vi "AlliGator Phasor Graph Actions.vi"(0 "AlliGator Q Elements in":T6[](array[typedef]), 1 "VI in":refnum<vi>, 2 "Script in":bool, 5 "Data Value Reference in":refnum<data-value>, 7 "AlliGator Q Event in":T7=enum."GUI:Idle", 9 "Data":variant, 11 "error in (no error)":errorcluster, 12 "AlliGator Ctrl Refnums":T8) -> (3 "Script out":bool, 4 "AlliGator Q Elements out":T6[](array[typedef]), 6 "Data Value Reference out":refnum<data-value>, 10 "[Notebook Message]":T1[](array[typedef]) {"Message Style"."Font Size" min=6.0 step=1.0}, 15 "error out":errorcluster)   [LabVIEW 2021, in "AlliGator Action Engine.lvlib"]
doc: "Processes AlliGator phasor graph-related actions."
uses:
  AlliGator Action Engine.lvlib
  Internal Variables/AlliGator Internal Variables v2.ctl
  <vilib>/vision/Image Controls.llb/IMAQ Image.ctl
  Internal Variables/AlliGator Gate Image Set.ctl
  Files/AlliGator FLI Dataset Type.ctl
  Files/AlliGator Data Series Type.ctl
  Dual-Channel Datasets/AlliGator Dataset Channel.ctl
  Settings/AlliGator Gate Arithmetic.ctl
  Source Image/AlliGator Displayed Image.ctl
  Image/Named ROI Description.ctl
  Phasor Graph/AlliGator Decay Metadata v3.ctl
  Decay Analysis/Decay Preprocessing/AlliGator Decay Background Subtraction Info.ctl
  Decay Analysis/Decay Preprocessing/AlliGator Baseline Subtraction Method.ctl
  Graphs/XY Graph/XY Graph Plot Shift Parameters.ctl
  Graphs/XY Graph/XY Graph Plot Shift Method.ctl
  Decay Analysis/Decay Preprocessing/AlliGator Decay Extrapolation Parameters.ctl
  Phasor/Calibration Phasor (m, phi).ctl
  Phasor/Phasor Reference Series.ctl
  Phasor/Phasor Calibration Map v2.ctl
  Phasor/Phasor (g, s).ctl
  Phasor Graph/AlliGator Raw Phasor Plot Data v5.ctl
  Phasor/Phasor Standard Deviation Options.ctl
  Phasor Plot/AlliGator Phasor Multi-Harmonic Data.ctl
  Phasor/Phasor Harmonic Data.ctl
  Decay Fit Parameter Map/AlliGator Decay Fit Options & Parameters v3.ctl
  Fits/IRF(X)PSED/Decay Fit Options v3.ctl
  Fits/Decay Convolution/Decay Model.ctl
  Fits/Residual Type.ctl
  Fits/IRF(X)PSED/Fit Weights Type.ctl
  Fits/Non-linear Fitting Method v2.ctl
  Fits/Fit Calculation Method.ctl
  Fits/Non-linear Fitting Algorithm.ctl
  Decay Analysis/Decay Fit/AlliGator Decay Fit Parameter Constraints 2.ctl
  Fits/IRF(X)PSED/Decay Fit Parameters In List.ctl
  Fits/IRF(X)PSED/MLE Baseline Offset Type.ctl
  Decay Analysis/Decay Preprocessing/AlliGator Decay Preprocessing Parameters.ctl
  Fits/IRF(X)PSED/Decay Fit Parameters & Derived Quantities List v2.ctl
  Fits/IRF(X)PSED/Decay Fit Result Constraint.ctl
  Decay Fit Parameter Map/AlliGator Parameter Maps Data.ctl
  AlliGator Q Event.ctl
  GUI/AlliGator Ctrl Refnums.ctl
  GUI/AlliGator Other Ctrl Refnums.ctl
  GUI/AlliGator State Indicator.ctl
  GUI/AlliGator Main Window Tabs.ctl
  GUI/AlliGator Phasor Plot Ctrl Refnums.ctl
  GUI/AlliGator Phasor Graph Ctrl Refnums.ctl
  Phasor/Phasor Calibration Type.ctl
  GUI/AlliGator Dataset Ctrl Refnums.ctl
  GUI/AlliGator Registered Events Ctrl Refnums.ctl
  GUI/AlliGator Image Histogram Control Refnums.ctl
  Histograms/Linear Histogram Options.ctl
  Histograms/Histogram Bin Option.ctl
  Histograms/Histogram Bin Position.ctl
  Decay Fit Parameter Map/AlliGator Decay Fit Map Control Refnums.ctl
  Parameter Map/AlliGator Parameter Map Control Refnums.ctl
  AlliGator Q Element.ctl
  Notebook/Notebook Message Object.ctl
  Rich Text Box/Text Formatting.ctl
  Rich Text Box/Text Colors.ctl
  Rich Text Box/Text Style.ctl
  Rich Text Box/Text Alignment.ctl
  Graphs/XY Graph/XY Graph Mouse Click Event Data.ctl
  Graphs/XY Graph/XY Graph Refnum.ctl
  <vilib>/Utility/miscctls.llb/LVPoint32TypeDef.ctl
  Graphs/XY Graph/XY Graph Selected Plot Info.ctl
  Phasor Graph/AlliGator Raw Phasor Plot Array Action.ctl
  Alligator Elements Order in Action Stack.ctl
  Rich Text Box/Text Format List.ctl
  Graphs/XY Graph/New Plot Information.ctl
  Graphs/Plot Scales.ctl
  Graphs/LabVIEW Plot Interpolation.ctl
  Graphs/Plot Point Style.ctl
  Globals, Variables, Constants/AlliGator Variables List.ctl
  Phasor Graph/AlliGator Phasor Plot Scatter Plot Parameters.ctl
  Phasor Graph/AlliGator Phasor Graph Parameter List.ctl
  Phasor Ratio/AlliGator Phasor Reference Data.ctl
  Phasor/Phasor (m, phi).ctl
  da8c548c-3fe3-4ac5-84e2-54aef6c91d4f.vi
  Graphs/Get Plot at Mouse Click (XY Graph)/Get Plot at Mouse Click [AAC].vi
  AlliGator Add Single Action to Stack.vi
  AlliGator Add Action Array to Stack.vi
  Variant/Variant to Data/Variant to Boolean.vi
  Variant/Variant to Data/Variant to Path.vi
  Variant/Variant to Data/Variant to [Path].vi
  Arrays/Signed Array Index.vi
  Variant/Variant to Data/Variant to I32.vi
  <vilib>/Utility/error.llb/Error Cluster From Error Code.vi
  Variant/Variant to Data/Variant to U32.vi
  <userlib>/_OpenG.lib/array/array.llb/Filter 1D Array with Scalar (I32)__ogtk.vi
  <vilib>/ErrorRing/Error Ring.xnode
  Graphs/Graphs.lvlib
  Variant/Variant to Data/Variant to Data.lvlib
  Phasor Graph/AlliGator Phasor Graph.lvlib
  Internal Variables/AlliGator Internal Variables.lvlib
  GUI/GUI.lvlib
  Phasor/Phasor.lvlib
  Graphs/XY Graph/XY Graph Add-Ons.lvlib
  Phasor Ratio/AlliGator Phasor Ratio.lvlib
  Strings/Strings.lvlib
  <userlib>/_OpenG.lib/array/array.llb/openg_array.lvlib
  Scripts/AlliGator Scripts.lvlib
  Source Image/AlliGator Source Image.lvlib
  Files/AlliGator Files.lvlib
  Settings/AlliGator Settings.lvlib
  Sound/Sound.lvlib
  Error/Error.lvlib
  Globals, Variables, Constants/AlliGator Globals, Variables & Constants.lvlib
  Phasor Calibration/AlliGator Phasor Calibration.lvlib
  Notebook/Notebook.lvlib
  Image/Image.lvlib
  Decay Analysis/Decay Preprocessing/AlliGator Decay Preprocessing.lvlib
  Phasor Plot/AlliGator Phasor Plot.lvlib
  Fits/Fits.lvlib
  Decay Analysis/Decay Fit/AlliGator Decay Fit.lvlib
  Decay Fit Parameter Map/AlliGator Decay Fit Parameter Map.lvlib
  GUI/AlliGator GUI.lvlib
  Rich Text Box/Rich Text Box.lvlib
  Dual-Channel Datasets/AlliGator Dual-Channel Datasets.lvlib
  Histograms/Histogram Window.lvlib
  Parameter Map/AlliGator Parameter Map.lvlib
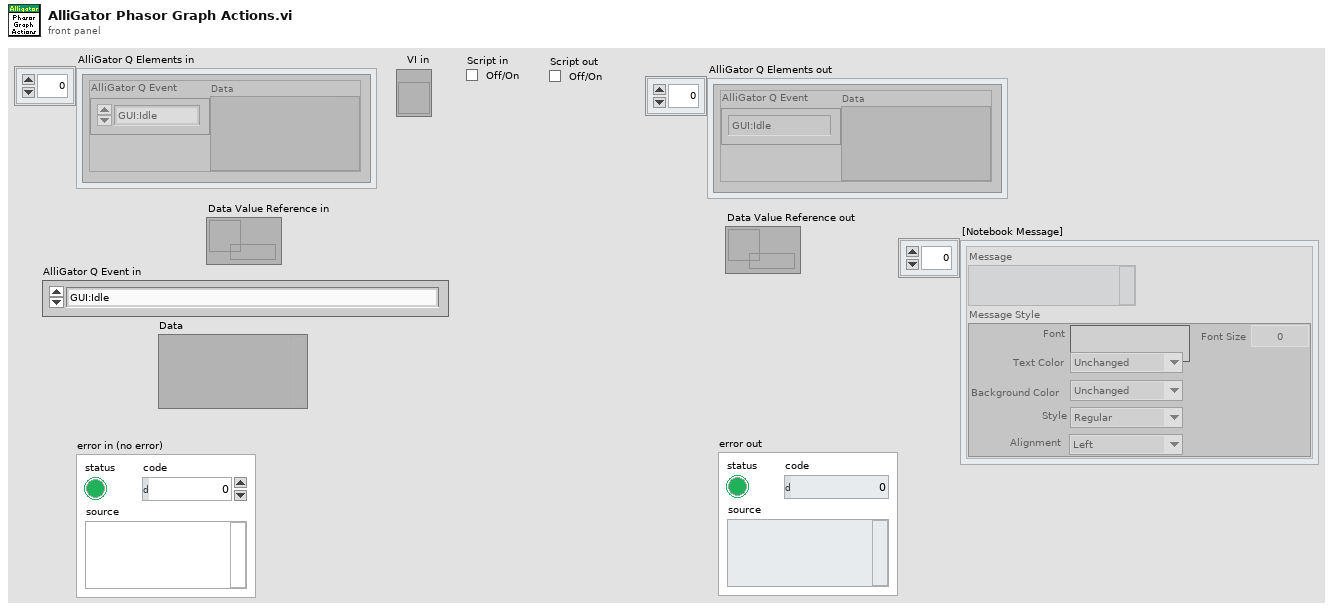
[diagram p1: front panel]
types:
  T1 = typedef "Notebook.lvlib/Notebook Message Object.ctl" = cluster{"Message":string, "Message Style":T2}
  T2 = typedef "Rich Text Box.lvlib/Text Formatting.ctl" = cluster{"Font":string, "Text Color":T3, "Background Color":T3, "Style":T4, "Font Size":dbl, "Alignment":T5}
  T3 = typedef "Rich Text Box.lvlib/Text Colors.ctl" = enum16{"Unchanged", "Black", "Blue", "Cyan", "Maroon", "Gray", "Violet", "Green", "Light Green", "Orange", "Yellow", "Magenta", "Red", "White"}
  T4 = typedef "Rich Text Box.lvlib/Text Style.ctl" = enum16{"Regular", "Bold", "Italic", "Underline", "Strikeout"}
  T5 = typedef "Rich Text Box.lvlib/Text Alignment.ctl" = enum16{"Left", "Right", "Center"}
  T6 = typedef "AlliGator Action Engine.lvlib/AlliGator Q Element.ctl" = cluster{"AlliGator Q Event":T7, "Data":variant}
  T7 = typedef "AlliGator Action Engine.lvlib/AlliGator Q Event.ctl" = enum16{"---- Files ----", "Files:Set Batch Export Files To Save", "Files:Set Dataset Loading & Pre-processing Options", "Files:Check #Frames in Dataset", "Files:Increment Frame Index", "Files:Open Mask Image", "Files:Open White Light Image", "Files:Open Single Dataset", "Files:New Folder of Folders Selected", "Files:Load File (all Types)_Scriptable", "Files:Move Flattened Series to Folders Series", "Files:Select Folder", "Files:Load FLI Dataset", "Files:Load Swiss SPAD 1 Dataset", "Files:Load Swiss SPAD 2 Dataset", "Files:Load .sdt FLI Dataset", "Files:Load .ptu FLI Dataset", "Files:Load .bin FLI Dataset", "Files:Load Single Gate Image Folder", "Files:Load I/m/phi Dataset (deprecated)", "Files:Load Single Image", "Files:Subtract Background File", "Files:Export FLI Dataset", "Files:Load HDF5 FLI Dataset", "Files:Set Destination File Path", "Files:Save Mask Image", "Files:Batch Conversion", "Files:New Folder Selected", "Files:Close FLI Dataset", "Files:Close FLI Dataset Series", "Files:Close White Light Image", "Files:Close Mask Image", "---- FLI Dataset ----", "FLI Dataset:Channel Arithmetic", "FLI Dataset:Export Average Lifetime Map as ASCII", "FLI Dataset:Export User-Defined Quantity Map as ASCII", "FLI Dataset:Python Function FLI Dataset Event", "FLI Dataset:ROI Analysis", "FLI Dataset:Tilted Logistic Square Gated IRF Characteristics Map", "FLI Dataset:Logistic Square Gated IRF Characteristics Map", "FLI Dataset:Square Gated IRF Characteristics Map", "FLI Dataset:Multi-ROI Single-Pixel Phasor Analysis", "FLI Dataset:Multi-ROI Single-Pixel NLSF Analysis", "FLI Dataset:All ROIs IRF Extraction", "FLI Dataset:All ROIs Decay Fit Non-Interactive (Fast + Individual IRF)", "FLI Dataset:All ROIs Phasor Analysis", "FLI Dataset:All ROIs Decay Fit", "FLI Dataset:Fluorescence Decay Statistics", "FLI Dataset:Update Decay Statistics Graph", "FLI Dataset:Get Decay from ROI", "FLI Dataset:All ROIs Average Lifetimes", "FLI Dataset:Save/Load Local IRFs", "FLI Dataset:Clear Local IRFs", "FLI Dataset:Phasor Calibration Maps (# Gates Series) Script", "FLI Dataset:Calibrated Phasor Map Series", "---- FLI Dataset Series ----", "FLI Dataset Series:Sum All Datasets in Series", "FLI Dataset Series:Add Dataset to Accumulated Dataset", "FLI Dataset Series:Display Accumulated Dataset", "FLI Dataset Series:Clear Dataset Series Sum", "FLI Dataset Series:Time-Series Analysis (NLSF)", "FLI Dataset Series:Time-Series Analysis (Phasor)", "---- Image ----", "Image:Update Image Profile Plots", "Image:Image Histogram Cursor Move", "Image:Image Histogram", "Image:Image Contrast", "Image:Set Image Histogram Cursor Move Flag", "Image:Clear Image Overlay", "Image:Use ROI as Search Area", "Image:Set ROI Diameter", "Image:Save Image Data as TIFF", "Image:Save Displayed Image with Overlay", "Image:Save Image Overlay Only", "Image:Save Image as Hot Pixel Mask", "Image:Change Source Image Color Palette", "Image:Copy Image to Clipboard", "Image:Source Image ROI Selection", "Image:Delete All ROIs", "Image:Delete All Unselected ROIs", "Image:Delete ROI", "Image:Merge All ROIs", "Image:Store ROI", "Image:Source Image ROI Storage", "Image:Export ROI Description to Notebook", "Image:Save ROI", "Image:Load ROI", "Image:Paste ROI Definition", "Image:Clear ROI", "Image:Identify ROIs in Mask Image", "Image:Create Complementary ROI", "Image:Create Contour ROI", "Image:Create ROI(s) from Pixels with Peak above Min_Scriptable", "Image:Create ROI(s) from Pixels with Intensity above Min_Scriptable", "Image:Compute ROI Statistics", "Image:Delete ROI(s) based on ROI Characteristics", "Image:Create ROI Grid", "Image:ROI to Individual Pixel ROIs", "Image:Python Function Source Image Event", "Image:Show Phasor Calibration Map ROI Centers", "Image:Convert ROI to Mask Image", "Image:Mouse Move", "Image:Mouse Up", "Image:Set Source Image Mouse Move Flag", "Image:Add Scale Bar Overlay", "Image:Delete Existing ROIs Option", "Image:Overlay ROI Median", "Image:Check Current ROI", "Image:Update True Pixel Value", "---- Decay ----", "Decay:Clear IRF/Reference Plot", "Decay:Add Decay to Graph", "Decay:Smoothen Plot", "Decay:Smoothen Plot Tail", "Decay:Average Selected Plots", "Decay:Extract IRF", "Decay:Optimal IRF Extraction", "Decay:Threshold IRF", "Decay:Fit to Model IRF", "Decay:Fit IRF to Square Gate", "Decay:Fit IRF to Logistic Square Gate", "Decay:Fit IRF to Tilted Logistic Square Gate", "Decay:Create Bounding Cursors Set", "Decay:Export Bounding Cursors Definition to Notebook", "Decay:Denoise Plot", "Decay:Compute Cumulative Function", "Decay:Use as Reference Decay", "Decay:Show Reference Decay/IRF", "Decay:Extrapolate Decay", "Decay:Create Head & Tail Bounding Cursors", "Decay:Store Cursor-defined Head & Tail Fractions", "Decay:Rebin Plot", "Decay:1-Normalize Decay", "Decay:[0-1]-Normalize Plot", "Decay:Straighten Decay", "Decay:Shift Decay", "Decay:Fold Decay", "Decay:Fit Decay", "Decay:Global Fit of Selected Decays", "Decay:Post Global Fit Script", "Decay:Add Global Fit Parameters to Graph", "Decay:Add Decay Parameter(s) to Plot (Graph)", "Decay:Export Decay to Phasor Graph", "Decay:Compute Average Lifetime", "Decay:Plot Convolution", "Decay:Graph Tip Strip Update", "---- Decay Statistics ----", "Decay Statistics:Tip Strip Update", "---- Intensity Time Trace ----", "Intensity Time Trace:Use File Timestamp", "Intensity Time Trace:Load Intensity Corrections File", "Intensity Time Trace:Clear Intensity Corrections File", "Intensity Time Trace:Tip Strip Update", "---- Phasor Plot ----", "Phasor Plot:Build Phasor Plot", "Phasor Plot:Change Phasor Plot Color Palette", "Phasor Plot:Adjust Phasor Plot Display Range", "Phasor Plot:Highlight Image ROI in Phasor Plot", "Phasor Plot:Save Phasor Plot Image with Overlay", "Phasor Plot:Export Complex Phasor Map", "Phasor Plot:Export Phasor Ratio Map", "Phasor Plot:Export Average Lifetime Map", "Phasor Plot:Compute Phase Lifetime Histogram", "Phasor Plot:Compute Phasor Ratio Histogram", "Phasor Plot:Compute Phase Lifetime vs Intensity Scatter Plot", "Phasor Plot:Weber 2-Component Decomposition", "Phasor Plot:Update Phasor Color Map Vertices", "Phasor Plot:Clear Phasor Overlay", "Phasor Plot:Use Segment Extremities as References", "Phasor Plot:Use UC/Segment Intersections as References", "Phasor Plot:Use UC/Principal Axis Intersections as References", "Phasor Plot:Use UC/Linear Fit Intersections as References", "Phasor Plot:Update Phasor Plot Reference", "Phasor Plot:Show Local Phasor Info in Phasor Plot", "Phasor Plot:Update Phasor Plot State", "Phasor Plot:Phasor Plot ROI Storage", "Phasor Plot:Phasor Plot ROI Selection", "Phasor Plot:Python Function Phasor Plot Event", "Phasor Plot:Overlay Phasor ROI, Ratio or Map in Source Image", "Phasor Plot:Compute Decay of Selected Phasors", "Phasor Plot:Phasor at Image Pixel", "Phasor Plot:Mouse Move", "Phasor Plot:Mouse Up", "Phasor Plot:Display Range Mouse Move", "Phasor Plot:Set Mouse Move Flag", "Phasor Plot:Update True Phasor Plot Value", "---- Phasor Graph ----", "Phasor Graph:Get Phasor Value", "Phasor Graph:Create New Phasor Plot Dialog", "Phasor Graph:Update Last Phasor Value", "Phasor Graph:Update Phasor (m, phi)", "Phasor Graph:Remove Single Phasor from Plot", "Phasor Graph:Add Single Phasor to Plot", "Phasor Graph:Remove Phasor Plot", "Phasor Graph:Remove Selected Phasor Plots", "Phasor Graph:Clear Phasor Data", "Phasor Graph:Clear Phasor Graph", "Phasor Graph:Cursor Move", "Phasor Graph:Draw Cursor Connecting Line", "Phasor Graph:Clear Cursor Connecting Line", "Phasor Graph:Find UC Intersection", "Phasor Graph:Use UC/Cursor-Defined Line Intersections", "Phasor Graph:Use Selected Plots Fitted Line/UC Intersections", "Phasor Graph:Use Selected Plots Principal Axis/UC Intersections", "Phasor Graph:Show Single Phasor", "Phasor Graph:Save Single Phasor Plot", "Phasor Graph:Save All Phasor Plots", "Phasor Graph:Load Phasor Plot(s)", "Phasor Graph:Phasor Multiplication", "Phasor Graph:Compute Average Phasor", "Phasor Graph:Compute Multiple Average Phasors (Selected Plots)", "Phasor Graph:Export Single Phasor Plot Phase Lifetimes", "Phasor Graph:Parameter 2 vs Parameter 1 Scatter Plot", "Phasor Graph:Use Cursor n Location", "Phasor Graph:Set Reference n to Current Phase Lifetime Value", "Phasor Graph:Set Reference n to Lifetime Value", "Phasor Graph:Set Cursor n Location", "Phasor Graph:Save Phasor Graph Image", "Phasor Graph:Update SEPL Plot", "Phasor Graph:Export Single Phasor Plot Data", "Phasor Graph:Export Selected Phasor Plots Data", "Phasor Graph:Python Function Phasor Graph Event", "Phasor Graph:Tip Strip Update", "---- Calibration ----", "Calibration:Set Calibration Type", "Calibration:Load/Save Phasor Calibration", "Calibration:Load/Save Phasor Calibration Series", "Calibration:Load/Save Phasor Calibration Map", "Calibration:Use as Calibration", "Calibration:Compute Optimal Calibration from Phasor References", "Calibration:Clear Phasor Calibration", "Calibration:Single Phasor Calibration Information", "Calibration:Use as Calibration Series", "Calibration:Use as Calibration Map", "Calibration:Clear Calibration Series", "Calibration:Phasor Calibration Series Information", "Calibration:Clear Calibration Map", "Calibration:Phasor Calibration Map Information", "Calibration:Apply Phasor Calibration", "Calibration:Update Single Plot Calibration", "Calibration:Update Multiple Plots Calibration", "Calibration:Clear Single Plot Calibration", "Calibration:Clear All Plots Calibrations", "Calibration:Clear Plot(s) Calibration(s)?", "---- Phasor Ratio ----", "Phasor Ratio:Clear Reference n", "Phasor Ratio:Toggle Selected Plot(s)  Lock to Reference 1", "Phasor Ratio:Use as Reference n", "Phasor Ratio:Send Reference n to Notebook", "Phasor Ratio:Toggle Selected Plot(s)  Lock to Reference 2", "Phasor Ratio:Compute Phasor Ratio at Mouse Location", "Phasor Ratio:Compute Phasor Plot's Average Phasor Ratio", "Phasor Ratio:Compute Time-Series Phasor Ratios", "Phasor Ratio:Fit Line to Phasor Ratio Plot", "Phasor Ratio:Save References", "Phasor Ratio:Load References", "Phasor Ratio:Update Phasor Reference 1", "Phasor Ratio:Update Phasor Reference 2", "Phasor Ratio:Move Cursor n to Reference n", "Phasor Ratio:Use as Phasor Reference 1 Lifetime", "Phasor Ratio:Use as Phasor Reference 2 Lifetime", "Phasor Ratio:Export Phasor Ratio Map as ASCII", "Phasor Ratio:Tip Strip Update", "---- Lifetime & Other Parameters Graph ----", "Lifetime:Compute Sliced Mean, SDV and CV Plots", "Lifetime:Plot Decay Shifts", "Lifetime:Plot Histogram", "---- Decay Fit Parameter Map ----", "Decay Fit Parameter Map:Export ROI NLSF Data as ASCII", "Decay Fit Parameter Map:Set Decay Fit Parameter Map Selection", "Decay Fit Parameter Map:Build Decay Fit Parameter Map", "Decay Fit Parameter Map:Change Decay Fit Parameter Map Color Palette", "Decay Fit Parameter Map:Export Decay Fit Parameter Map Data as ASCII", "Decay Fit Parameter Map:Export All Decay Fit Parameter Maps Data as ASCII", "Decay Fit Parameter Map:Selected Parameter Scatterplot", "Decay Fit Parameter Map:Parameter 2 vs Parameter 1 Scatterplot", "Decay Fit Parameter Map:Save Decay Fit Parameter Map Image", "Decay Fit Parameter Map:Save-Load IRFs & Fit Data", "Decay Fit Parameter Map:Update Local Decay Plots", "Decay Fit Parameter Map:Python Function Decay Fit Parameters Map Event", "Decay Fit Parameter Map:Overlay Decay Fit Parameter Map in Source Image", "Decay Fit Parameter Map:Selected Parameter vs Intensity Scatterplot", "Decay Fit Parameter Map:Mouse Up", "Decay Fit Parameter Map:Mouse Move", "Decay Fit Parameter Map:Display Range Mouse Move", "Decay Fit Parameter Map:Change Map Resolution", "Decay Fit Parameter Map:Variance Significance Maps", "Decay Fit Parameter Map:Fit Result Constraints Window", "---- Parameter Map ----", "Parameter Map:Export ROI Parameters Data as ASCII", "Parameter Map:Delete Parameter Map Set", "Parameter Map:Update Parameter List", "Parameter Map:Build Parameter Map", "Parameter Map:Change Parameter Map Color Palette", "Parameter Map:Export Parameter Map Data as ASCII", "Parameter Map:Export All Parameter Maps Data as ASCII", "Parameter Map:Selected Parameter Scatterplot", "Parameter Map:Parameter 2 vs Parameter 1 Scatterplot", "Parameter Map:Selected Parameter vs Intensity Scatterplot", "Parameter Map:Save Parameter Map Image", "Parameter Map:Save-Load IRFs & Parameter Maps (TODO)", "Parameter Map:Set Parameter Map Selection", "Parameter Map:Python Function Parameter Map Event", "Parameter Map:Overlay Parameter Map in Source Image", "Parameter Map:Update Local Decay Plots", "Parameter Map:Mouse Up", "Parameter Map:Mouse Move", "Parameter Map:Display Range Mouse Move", "---- Generic Graph ----", "Generic Graph:Generic XY Graph Event", "Generic Graph:Python Function XY Graph Event", "Generic Graph:New Plot", "Generic Graph:Save Plot", "Generic Graph:XY Plot Histogram", "Generic Graph:Set XY Graph Plot Name", "Generic Graph:Set Last Cursor Style", "Generic Graph:Tip Strip Update", "---- GUI ----", "GUI:Start Script", "GUI:Type of Displayed Image Changed", "GUI:Gate Image Slide Changed", "GUI:Show Busy Icon", "GUI:Show Busy Icon & Abort Button", "GUI:Hide Busy Icon", "GUI:Hide Busy Icon & Abort Button", "GUI:Abort", "GUI:End Script", "GUI:Start Timing", "GUI:End Timing", "GUI:Set State Indicator", "GUI:Send Parameters JSON Strings to Clipboard", "GUI:Set Gate Step", "GUI:Idle", "GUI:Initialization", "GUI:Quit", "GUI:Increment Dataset Index", "GUI:Set Dataset Index to -1", "GUI:Time Series Slider Moved", "GUI:Time Series Slider Changed", "GUI:Toggle Playback or Loop", "GUI:Playback Script", "GUI:Set Phasor Frequency", "GUI:Open Window", "GUI:Start Test Script", "GUI:End Test Script", "GUI:Set Verbose Mode", "GUI:Set Verbose Settings Mode", "DEBUG"}
  T8 = typedef "AlliGator GUI.lvlib/AlliGator Ctrl Refnums.ctl" = cluster{"Other AlliGator Ctrl Refnums":T9, "Phasor Plot Ctrl Refnums":T10, "Phasor Graph Ctrl Refnums":T11, "Dataset Control Refnums":T12, "Registered Events Ctrl Refnums":T13, "Image Histogram Ctrl Refnums":T14, "Decay Fit Map Ctrl Refnums":T15, "Parameter Map Ctrl Refnums":T16}
  T9 = typedef "AlliGator GUI.lvlib/AlliGator Other Ctrl Refnums.ctl" = cluster{"State Indicators":refnum<vi>, " Progress Bar":refnum<vi>, "Decay Graph Active":refnum<vi>, "Decay Statistics Bin":refnum<vi>, "Time Step":refnum<vi>, "Use File Timestamp":refnum<vi>, "Tab Control":refnum<vi>, "CPU":refnum<vi>, "Abort Fit":refnum<vi>, "Dataset File/Folder Path":refnum<vi>, "Abort ROI Creation":refnum<vi>, "Event LED":refnum<vi>, "Dataset File/Folder Path 2":refnum<vi>, "Dataset File/Folder Path 3":refnum<vi>, "Dataset File/Folder Path 4":refnum<vi>, "Dataset File/Folder Path 5":refnum<vi>, "Dataset File/Folder Path 6":refnum<vi>, "Dataset File/Folder Path 7":refnum<vi>, "Dataset File/Folder Path 8":refnum<vi>, "Dataset File/Folder Path 9":refnum<vi>, "Dataset File/Folder Path 10":refnum<vi>, "Dataset File/Folder Path 11":refnum<vi>}
  T10 = typedef "AlliGator GUI.lvlib/AlliGator Phasor Plot Ctrl Refnums.ctl" = cluster{"Phasor Ratio":refnum<vi>, "Modulus Lifetime":refnum<vi>, "Phasor at cursor (m, phi)":refnum<vi>, "Phase Lifetime":refnum<vi>, "Phasor at cursor (g, s)":refnum<vi>, "Phasor Plor Average Lifetime":refnum<vi>, "Phasor Plot Active":refnum<vi>, "Save Phasor Plot":refnum<vi>, "Image Overlay Color":refnum<vi>, "Phasor Plot Color Scale":refnum<vi>, "Reference 1 Button":refnum<vi>, "Reference 2 Button":refnum<vi>, "True Phasor Plot Value":refnum<vi>}
  T11 = typedef "AlliGator GUI.lvlib/AlliGator Phasor Graph Ctrl Refnums.ctl" = cluster{"Phasor Ratio":refnum<vi>, "Modulus Lifetime":refnum<vi>, "Phasor at cursor (m, phi)":refnum<vi>, "Phase Lifetime":refnum<vi>, "Phasor at cursor (g, s)":refnum<vi>, "Phasor Graph Average Lifetime":refnum<vi>, "Phasor Graph Active":refnum<vi>, "Save Phasor Graph":refnum<vi>, "Phasor Frame Slide":refnum<vi>, "Single Step Phasor":refnum<vi>, "Calibration Type":refnum<vi>, "Show Line":refnum<vi>, "Phase Lifetime 1":refnum<vi>, "Phase Lifetime 2":refnum<vi>, "Phasor Graph Frequency":refnum<vi>, "Phasor Reference 1 Control":refnum<vi>, "Phasor Reference 2 Control":refnum<vi>, "Calibration Lifetime":refnum<vi>, "Phase Lifetime SDV":refnum<vi>, "Average Lifetime SDV":refnum<vi>, "Phasor Ratio SDV":refnum<vi>, "Modulus Lifetime SDV":refnum<vi>}
  T12 = typedef "AlliGator GUI.lvlib/AlliGator Dataset Ctrl Refnums.ctl" = cluster{"Current Data":refnum<vi>, "Gate Image Slide":refnum<vi>, "Time Point Slide":refnum<vi>, "Current Time Stamp":refnum<vi>, "Save Image":refnum<vi>, "Displayed Image":refnum<vi>, "Overlay Mode":refnum<vi>, "Phasor Overlay Color":refnum<vi>, "Image Color Scale":refnum<vi>, "Use ROI as Search Area":refnum<vi>, "Source Image ROI Color":refnum<vi>, "True Pixel Value":refnum<vi>}
  T13 = typedef "AlliGator GUI.lvlib/AlliGator Registered Events Ctrl Refnums.ctl" = cluster{"Time Point Slider":refnum<vi>, "Phasor Plot Display Range":refnum<vi>, "Decay Graph":refnum<vi>, "Decay Statistics Graph":refnum<vi>, "Intensity Time Trace":refnum<vi>, "Phasor Graph":refnum<vi>, "Phasor Ratio Graph":refnum<vi>, "Lifetime Graph":refnum<vi>, "Phasor Plot Display":refnum<vi>, "Source Image Display":refnum<vi>, "Decay Fit Parameter Map Display Range":refnum<vi>, "Decay Fit Parameter Map Display":refnum<vi>, "Parameter Map Display Range":refnum<vi>, "Parameter Map Display":refnum<vi>, "Phasor Plot Display Range":refnum<vi>}
  T14 = typedef "AlliGator GUI.lvlib/AlliGator Image Histogram Control Refnums.ctl" = cluster{"Image Histogram":refnum<vi>, "Image Histogram Options":refnum<vi>, "Image Histogram Active":refnum<vi>, "Image Histogram Upper Percentile":refnum<vi>, "Image Histogram Lower Percentile":refnum<vi>, "Auto-Adjust Contrast":refnum<vi>}
  T15 = typedef "AlliGator Decay Fit Parameter Map.lvlib/AlliGator Decay Fit Map Control Refnums.ctl" = cluster{"Decay Fit Parameter Map Color Scale":refnum<vi>, "Decay Fit Parameter":refnum<vi>, "Max Parameter":refnum<vi>, "Min Parameter":refnum<vi>, "Decay Fit Parameter Map Display":refnum<vi>, "Decay Fit Parameter Map Display Range":refnum<vi>, "Decay Parameter Map X":refnum<vi>, "Decay Parameter Map Y":refnum<vi>, "Decay Parameter Map Value":refnum<vi>}
  T16 = typedef "AlliGator Parameter Map.lvlib/AlliGator Parameter Map Control Refnums.ctl" = cluster{"Parameter Map Color Scale":refnum<vi>, "Map Parameter":refnum<vi>, "Max Parameter":refnum<vi>, "Min Parameter":refnum<vi>, "Parameter Map Display":refnum<vi>, "Parameter Map Display Range":refnum<vi>, "Parameter Map Set":refnum<vi>, "Parameter Map X":refnum<vi>, "Parameter Map Y":refnum<vi>, "Parameter Map Value":refnum<vi>}
  T17 = typedef "XY Graph Add-Ons.lvlib/XY Graph Selected Plot Info.ctl" = cluster{"Multiplot XY Graph":T18, "Mouse Coordinates":T19, "Plot Index":i32}
  T18 = typedef "XY Graph Add-Ons.lvlib/XY Graph Refnum.ctl" = refnum<vi>
  T19 = typedef "LVPoint32TypeDef.ctl" = cluster{"Horizontal":i32, "Vertical":i32}
  T20 = typedef "XY Graph Add-Ons.lvlib/XY Graph Mouse Click Event Data.ctl" = cluster{"Multiplot XY Graph":T18, "Mouse Coordinates":T19}
  T21 = typedef "Phasor.lvlib/Calibration Phasor (m, phi).ctl" = cluster{"m":dbl, "phi":dbl, "Phasor Frequency":dbl[unit], "Reference Lifetime":dbl[unit]}
  T22 = typedef "Phasor.lvlib/Phasor (g, s).ctl" = cluster{"g":dbl, "s":dbl}
  T23 = typedef "AlliGator Phasor Graph.lvlib/AlliGator Raw Phasor Plot Array Action.ctl" = enum16{"Clear All", "-", "Add Raw Phasor Plot", "Delete Raw Phasor Plot", "Replace Raw Phasor Plot", "---------------------", "Add Phasor to Plot", "Replace Phasor in Plot", "Remove Phasor in Plot"}
  T24 = typedef "Notebook.lvlib/Text Format List.ctl" = enum16{"Message", "Result", "Error", "Setting", "Verbose", "Warning"}
  T25 = typedef "AlliGator Action Engine.lvlib/Alligator Elements Order in Action Stack.ctl" = enum16{"Enqueue 2 AFTER 1", "Enqueue 2 BEFORE 1"}
  T26 = typedef "XY Graph Add-Ons.lvlib/New Plot Information.ctl" = cluster{"Multiplot XY Graph":refnum<vi>, "Plot Name":string, "Plot Scales":T27, "Plot Interpolation":T28, "Point Style":T29, "Plot Color":u32, "Plot Metadata":variant}
  T27 = typedef "XY Graph Add-Ons.lvlib/Plot Scales.ctl" = cluster{"X Scale":u32, "Y Scale":u32}
  T28 = typedef "Graphs.lvlib/LabVIEW Plot Interpolation.ctl" = enum16{"Point (.)", "Stepwise Right (--.)", "Line + Point (\\. /)", "Stepwise Left (.--)", "Stepwise Centered (-.-)", "Stepwise Vertical (|.|)", "Line (-)", "Use Previous Plot's Style"}
  T29 = typedef "Graphs.lvlib/Plot Point Style.ctl" = enum16{"not defined", "None", "Empty Circle", "Filled Circle", "Thick Circle", "Dotted Circle", "Empty Square", "Filled Square", "Thick Square", "Dotted Square", "Small Filled Square", "Dot", "Cross", "Tiny Cross", "Large X", "Small x", "Diamond", "Small Empty Square"}
  T30 = typedef "AlliGator Globals, Variables & Constants.lvlib/AlliGator Variables List.ctl" = enum16{"---- GUI ----", "GUI:Initialization Status", "GUI:State Indicators Refnum", "GUI:Original AlliGator Menu Items", "GUI:Current Action Loop State", "GUI:Script in progress", "GUI:Playback", "GUI:Loop Playback", "GUI:Search ROI Used", "GUI:Search ROI", "Decay Graph Max Legend Size", "Intensity Graph Max Legend Size", "Decay Statistics Graph Max Legend Size", "Phasor Graph Max Legend Size", "Phasor Ratio Graph Max Legend Size", "Lifetime Graph Max Legend Size", "---- Files ----", "Files:Export Dataset Frames as Individual Files", "Files:Show Batch Export Help Balloons", "Files:Frames in Dataset", "Files:ptu File Frame Start Indices", "Files:Current Frame in Dataset", "Files:Current Frame Timestamp", "Files:Dataset Loaded", "Files:Dataset Metadata", "Files:Dataset Channel", "Files:Dataset Data Description", "Files:Background Dataset Metadata", "Files:Background Dataset Channel", "Files:Background Dataset Data Description", "Files:Background File Subtraction", "Files:Background File Path", "Files:Background File Pile-up Correction", "Files:Background File Pixel Well Capacity", "Files:Background File Scaling Factor", "Files:Current Dataset Load Settings", "Files:Dataset Path", "Files:ICCD-specific Information", "Files:Macrotime Gate Separation", "------ Python Plugins ------", "Python Plugins:Information", "Python Plugins:Python Session", "Python Plugins:Valid Python Session?", "---- Source Image ----", "Source Image:ROIs", "Source Image:Current ROI", "Source Image:ROI Event Refnum", "X_Source Image:Display Range", "X_Source Image:Palette Information", "X_Source Image:Type of Displayed Image", "X_Time Gate Slider", "Source Image:Palette List", "Source Image:Scale", "Source Image:ROI Overlay Color", "Source Image:Overlay to Erase", "Source Image:Is Displayed Image Accumulated", "Source Image:White Light Image Modified", "Source Image:Mask Image Modified", "---- Image Profile Window ----", "Image Profile:Window Event Refnum", "Image Profile:IntensityType", "Image Profile:Intensity Average Type", "Image Profile:Intensity-weighted SDV", "Image Profile:Box Profile Type", "Image Profile:Window Open", "Image Profile:Plotted Fit Parameter", "------ Phasor Graph -------", "Phasor Graph:Show Line", "---- Phasor Plot ---", "Phasor Plot:Parameters Changed", "Phasor Plot:FLI Dataset Modified since last Calculation", "Phasor Harmonics Data", "Selected Phasor Harmonics", "Phasor Harmonic Manager Event Refnum", "Phasor Plot:ROIs", "Phasor Plot:Current ROI", "Phasor Plot:ROI Event Refnum", "Phasor Plot:Image Reference Points", "Phasor Plot:Computed", "Phasor Plot:Palette Information", "Phasor Plot:Palette List", "Phasor Plot:Phasor Ratio Palette Information", "Phasor Plot:Phasor Ratio Palette List", "Phasor Plot:Image Scale", "Phasor Plot:Image Overlay to Erase", "Phasor Plot:Image Elements to Update", "Phasor Plot:Current Calculation Parameters", "Phasor Plot:Current Calibration Options", "Phasor Plot:Reset Cumulated Phasor Plot", "Phasor Plot:Reference 1", "Phasor Plot:Lifetime Reference 1", "Phasor Plot:Reference 1 Frequency", "Phasor Plot:Reference 2", "Phasor Plot:Lifetime Reference 2", "Phasor Plot:Reference 2 Frequency", "---- Decay Analysis ----", "Number of Selected Decays to Fit", "LS Fit Results", "LAR Fit Results", "BS Fit Results", "Last Decay Max - Min", "Best Fit Parameters", "Best Fit Parameter Names", "Actual Size X", "Actual Size Y", "Binning X", "Binning Y", "Actual # Gates", "Dataset Number", "Gates to...", "Gates Skipped", "Gates to keep", "Gate Step", "Gate Separation", "Reversed Gates", "Pile-up Correction", "Pixel Well Capacity", "Background Subtracted", "Background Subtraction Method", "Background Definition Range", "Background File (deprecated)", "Number of Dataset Accumulated", "Array of Accumulated Dataset Paths", "Do Averaged Datasets", "Destination File Path", "Process Plot Target", "Use 1/D as Phasor Frequency", "---- Decay Fit Parameter Map -----", "Decay Fit Parameter Map:Palette Information", "Decay Fit Parameter Map:Palette List", "Decay Fit Parameter Map:X Resolution", "Decay Fit Parameter Map:Y Resolution", "Decay Fit Parameter Map:Use Decay Fit Result Constraints", "Decay Fit Parameter Map:Decay Fit Result Constraints", "Decay Fit Parameter Map:Decay Fit Result Constraints Applied", "---- Parameter Map ----", "Parameter Map:Palette Information", "Parameter Map:Palette List", "------- Local Decay Window ---------", "Local Decay Graph Window:Event Refnum", "Local Decay Graph Window:Use normalized IRF for convolution", "----- Miscellaneous ----", "Misc:Skippable Dialog Windows Status"}
  T31 = cluster{"Mouse Click Event Data":T20, "Save as...":bool}
  T32 = typedef "AlliGator Phasor Graph.lvlib/AlliGator Phasor Plot Scatter Plot Parameters.ctl" = cluster{"Parameter 2":T33, "Parameter 1":T33}
  T33 = typedef "AlliGator Phasor Graph.lvlib/AlliGator Phasor Graph Parameter List.ctl" = enum16{"Time Stamp", "Index", "Phasor Parameters", "Phasor g", "Phasor s", "Phasor phi", "Phasor m", "Modulus Lifetime", "Phase Lifetime", "ROI Parameters", "ROI Center x", "ROI Center y", "ROI # pixels ", "Decay Parameters", "Intensity", "Background/Gate", "Intensity - Background", "Fitted Lifetime", "Fitted Intensity", "Phasor Ratio Parameters", "Amplitude Phasor Ratio", "Intensity Phasor Ratio", "Amplitude-Averaged Lifetime", "Intensity-Averaged Lifetime", "-", "Phasor Parameters SDV", "Phasor g SDV", "Phasor s SDV", "Phasor phi SDV", "Phasor m SDV", "Phase Lifetime SDV", "Modulus Lifetime SDV", "Phasor Ratio Parameters SDV", "Amplitude Phasor Ratio SDV", "Intensity Phasor Ratio SDV", "Amplitude-Averaged Lifetime SDV", "Intensity-Averaged Lifetime SDV"}
  T34 = cluster{"Current Phasor (g, s)":T22, "Cursor Id":u32}
  T35 = typedef "AlliGator Phasor Ratio.lvlib/AlliGator Phasor Reference Data.ctl" = cluster{"Data Type":string, "Data":variant}
  T36 = typedef "Phasor.lvlib/Phasor (m, phi).ctl" = cluster{"m":dbl, "phi":dbl}
  T37 = typedef "AlliGator Internal Variables.lvlib/AlliGator Internal Variables v2.ctl" = cluster{"----------------------------- Images -----------------------------":u8, "Displayed Image":T38, "White Light Image":T38, "Mask Image":T38, "ROI Mask Image":T38, "Current Dataset Images 1":T39, "Background Dataset Images 1":T39, "Current Dataset Images 2":T39, "Background Dataset Images 2":T39, "Current Dataset Arithmetic Images":T39, "Accumulated Dataset Images 1":T39, "Accumulated Dataset Images 2":T39, "Accumulated Dataset Arithmetic Images":T39, "----------------------------- File Paths -----------------------------":u8, "Phasor Plot Image":T38, "Decay Fit Parameter Map Image":T38, "Parameter Map Image":T38, "Single Data Point Path":path, "White Light Image Path":path, "Mask Image Path":path, "Time-Series Folder":path, "[Time-Series Paths]":path[], "----------------------------- FLI Dataset -----------------------------":u8, "Current Dataset":i32, "Single Dataset Type":T40, "Current Folder":string, "AlliGator Data Series Type":T41, "# Datasets":i32, "Dual-Channel Dataset":bool, "Selected Channel Name":string, "Dataset Channel":T42, "Channel Arithmetic":T43, "Dual-Channel Background Dataset":bool, "Background Channel":T42, "Dual-Channel Accumulated Dataset":bool, "Start Time":dbl, "[Time-Series Timestamps]":dbl[], "[Intensity Corrections]":dbl[], "Time Series Script":bool, "Type of Displayed Image":T44, "Gate Image Slide":u16, "# Gates":i32, "ROIs":T45[], "----------------------------- Decays -----------------------------":u8, "ROI Decay":cluster{"t Array":dbl[], "I Array":dbl[]}, "Valid Decay":bool, "Decay  Metadata":T47, "Reference Decay Plot Name":string, "Reference Decay":cluster{"t Array":dbl[], "I Array":dbl[]}, "Decay Shift Plot":cluster{"Time Stamps":dbl[], "Decay Shifts":dbl[]}, "[Decays Max Values]":sgl[], "[Decays Min Values]":sgl[], "----------------------------- Calibration -----------------------------":u8, "Calibration Phasor":T21, "Calibration Phasor Series":T53, "Phasor Calibration Map":T54, "Calibration Map MD5 Digest":string, "----------------------------- Phasor Graph -----------------------------":u8, "Last Raw Phasor":T22, "Last Calibrated Phasor":T22, "Last Calibrated Phasor SDV":T22, "Phasor Graph:Phasor Plot":cluster{"g Array":dbl[], "s Array":dbl[]}, "Phasor Graph:Phasor SDV Plot":cluster{"g Array":dbl[], "s Array":dbl[]}, "[Phasor Graph:Raw Phasor Plots]":T55[], "Phasor Plot locked to Ref 1":i32, "[Phasor Plot(s) locked to Ref 1]":i32[], "[Phasor Plot(s) locked to Ref 2]":i32[], "[Pixel Phasors]":T22[], "----------------------------- Phasor Plot -----------------------------":u8, "[[Sum Image]]":dbl[][], "[[CSG Phasors]]":csg[][], "[[Valid Pixel?]]":bool[][], "[[Phasor Ratios]]":dbl[][], "[[Average Lifetimes]]":dbl[][], "Amplitude Weighted Average Lifetime":bool, "I/m/phi Dataset":cluster{"I/m/phi Dataset?":bool, "Base Frequency":dbl[unit], "Harmonic Orders":u8[]}, "Multi Phasor Plot Data":T57, "----------------------------- Decay Fit Parameter Map -----------------------------":u8, "Decay Fit Options & Parameters":T59, "Fit Options: Decay Preprocessing Parameters":T70, "Fit Options: Reference Decay":cluster{"t Array":dbl[], "I Array":dbl[]}, "Is Full Image Parameters Map":bool, "Is Single-Pixels Parameters Map":bool, "NLSF Parameters Map X Resolution":i32, "NLSF Parameters Map Y Resolution":i32, "[Single Decay Fit Parameters]":dbl[], "Fit Model":T61, "[[Multiple Decays Fit Parameters]]":dbl[][], "[[Multiple Decays Fit Parameter SDVs]]":dbl[][], "[[IRFs]]":dbl[][], "[ROI Descriptors]":T46[], "IRF Array Time Axis":dbl[], "Decay Array Time Axis":dbl[], "[Decay Fit Parameter Names]":T71[], "[Decay Sum]":dbl[], "Array of Decay Fit Result Constraints":T72[], "Selected ROIs Array":bool[], "----------------------------- Parameter Maps -----------------------------":u8, "[Map Set Names]":string[], "[Parameter Maps]":T73[], "[[User-defined Quantities]]":dbl[][], "User-defined Quantity":string}
  T38 = typedef "IMAQ Image.ctl" = refnum<image>
  T39 = typedef "AlliGator Internal Variables.lvlib/AlliGator Gate Image Set.ctl" = cluster{"SGL Image Max":T38, "SGL Image Sum":T38, "SGL Gate Images":T38[], "SGL Image Min":T38}
  T40 = typedef "AlliGator Files.lvlib/AlliGator FLI Dataset Type.ctl" = enum16{"HDF5 FLI Dataset", "Gate Image Folder", ".sdt FLI Dataset (Becker & Hickl)", ".ptu FLI Dataset (PicoQuant)", "SS1 FLI Dataset", "SS2 FLI Dataset", "I/m/phi Dataset", ".bin FLI Dataset (PicoQuant Binned)", ".bin FLI Dataset (Piccolo Binned)", ".mat FLI Dataset"}
  T41 = typedef "AlliGator Files.lvlib/AlliGator Data Series Type.ctl" = enum16{"Not a Supported Series", "Gate Images Folder Series", "SwissSPAD 2 Dataset Series", "B&H FLI Dataset Series", "PicoQuant PTU FLI Dataset Series", "PicoQuant BIN FLI Dataset Series", "Piccolo hist BIN FLI Dataset Series", "HDF5 FLI Dataset Series"}
  T42 = typedef "AlliGator Dual-Channel Datasets.lvlib/AlliGator Dataset Channel.ctl" = enum16{"G2", "INT"}
  T43 = typedef "AlliGator Settings.lvlib/AlliGator Gate Arithmetic.ctl" = enum16{"None", "INT-G2", "G2/INT*<INT>", "(1 - G2/INT)*<INT>"}
  T44 = typedef "AlliGator Source Image.lvlib/AlliGator Displayed Image.ctl" = enum16{"Single Gate", "Sum of All Gates", "Max of All Gates", "Min of All Gates", "-", "White Ligth Image", "Mask Image"}
  T45 = typedef "Image.lvlib/Named ROI Description.ctl" = cluster{"ROI Descriptor":T46, "ROI Name":string, "Overlay Color":u32}
  T46 = typedef "ROI Descriptor" = cluster{"Global Rectangle":i32[], "Contours":cluster{"ID":enum32{"External", "Internal"}, "Type":u32, "Coordinates":i32[]}[]}
  T47 = typedef "AlliGator Phasor Graph.lvlib/AlliGator Decay Metadata v3.ctl" = cluster{"ROI Descriptor":T46, "ROI Center":cluster{"X":i32, "Y":i32}, "Decay Background Subtraction Info":T48, "Decay Reverted":bool, "Decay Smoothened":bool, "Decay Straightened":bool, "Fitted Tau (Decay Straightening)":dbl, "Decay Shift Parameters":T50, "Decay Shifted":bool, "Decay Extrapolated":bool, "Decay Extrapolation Parameters":T52, "Decay Normalized":bool, "Fold Decay":bool, "# Folds":u32}
  T48 = typedef "AlliGator Decay Preprocessing.lvlib/AlliGator Decay Background Subtraction Info.ctl" = cluster{"Laser Period":dbl[unit], "Gate Duration":dbl[unit], "Baseline Subtraction Method":T49, "Background Definition Range":cluster{"Min Gate":dbl[unit], "Max Gate":dbl[unit]}, "Total Intensity w/o Bkgd Subtraction":dbl, "Bkgd-subtracted Intensity (exp)":dbl, "# Data Points":i32, "Background/Gate":dbl, "Fitted Lifetime":dbl[unit], "Bkgd-subtracted Intensity (theo)":dbl}
  T49 = typedef "AlliGator Decay Preprocessing.lvlib/AlliGator Baseline Subtraction Method.ctl" = enum16{"Mean", "Min", "Square Gated Single-Exponential", "File", "Constant"}
  T50 = typedef "XY Graph Add-Ons.lvlib/XY Graph Plot Shift Parameters.ctl" = cluster{"Type":T51, "Shift":dbl[unit], "Threshold":dbl, "Rotate":bool}
  T51 = typedef "XY Graph Add-Ons.lvlib/XY Graph Plot Shift Method.ctl" = enum16{"Default", "CFD", "Threshold", "Cross-Correlation"}
  T52 = typedef "AlliGator Decay Preprocessing.lvlib/AlliGator Decay Extrapolation Parameters.ctl" = cluster{"Additional Points":u32, "Head Fraction":dbl, "Fitted Tau":dbl, "Use Periodicity":bool, "Use Cursors":bool, "Tail Fraction":dbl}
  T53 = typedef "Phasor.lvlib/Phasor Reference Series.ctl" = cluster{"m Array":dbl[], "phi Array":dbl[], "Phasor Frequency":dbl[unit], "Calibration Lifetime":dbl[unit]}
  T54 = typedef "Phasor.lvlib/Phasor Calibration Map v2.ctl" = cluster{"Phasor Frequency":dbl[unit], "Calibration Lifetime":dbl[unit], "ROI Centers":cluster{"X":i32, "Y":i32}[], "ROI Descriptors":T46[], "Map Resolution X":i32, "Map Resolution Y":i32, "z Array":cdb[]}
  T55 = typedef "AlliGator Phasor Graph.lvlib/AlliGator Raw Phasor Plot Data v5.ctl" = cluster{"Phasor Plot Name":string, "Raw Phasor Plot":T22[], "Phasor Frequency":dbl[unit], "[Decay Metadata]":T47[], "Raw Phasor Plot SDV":T22[], "Phasor SDV Options":T56, "[Calibration Phasor]":T21[], "Intensity Array":dbl[]}
  T56 = typedef "Phasor.lvlib/Phasor Standard Deviation Options.ctl" = cluster{"Compute Estimated SDV":bool, "# Replicas":u32, "Use Estimated Average Phasor":bool}
  T57 = typedef "AlliGator Phasor Plot.lvlib/AlliGator Phasor Multi-Harmonic Data.ctl" = cluster{"Base Frequency":dbl[unit], "# Harmonics":u8, "Harmonic Orders":u8[], "Phasor Plot Settings Checksum":u64, "Phasor Harmonic Data Array":T58[]}
  T58 = typedef "Phasor.lvlib/Phasor Harmonic Data.ctl" = cluster{"Phasor Harmonic Name":string, "Phasor Plot Settings Checksum":u64, "Phasor Frequency":dbl[unit], "Base Frequency":dbl[unit], "Harmonic Order":u8, "Phasor Plot Parameters":string, "Phasor Array [[CSG]]":csg[][], "Dataset File Path":path}
  T59 = typedef "AlliGator Decay Fit Parameter Map.lvlib/AlliGator Decay Fit Options & Parameters v3.ctl" = cluster{"SYNC Period":dbl[unit], "Fit Options":T60, "Fit Parameter Constraints":T67[], "MLE Baseline Offset":dbl, "MLE Baseline Offset Type":T69}
  T60 = typedef "Fits.lvlib/Decay Fit Options v3.ctl" = cluster{"Show Fit Residuals":bool, "Fit Model":T61, "Residual Type":T62, "Max Decay Percentile":dbl, "Min Decay Percentile":dbl, "Show Full Decay":bool, "Weights":T63, "Fitting Method":T64, "Compute Parameter Uncertainties":bool, "Periodic Boundaries":bool, "Model Calculation":T65, "Period":dbl[unit], "Termination Criteria":cluster{"Max Iterations":i32, "Max Function Calls":i32, "Max Time":dbl[unit], "Function Tolerance":dbl, "Parameter Tolerance":dbl, "Gradient Tolerance":dbl, "Min Lambda":dbl, "Max Lambda":dbl, "Initial Tick Count":u32}, "Offset Resolution":dbl[unit], "Use Local IRF":bool, "Fitting Algorithm":T66, "Show Confidence Interval ":bool, "Confidence Level":dbl}
  T61 = typedef "Fits.lvlib/Decay Model.ctl" = enum16{"1-Exponential", "2-Exponentials"}
  T62 = typedef "Fits.lvlib/Residual Type.ctl" = enum16{"Standard", "Normalized", "Reduced"}
  T63 = typedef "Fits.lvlib/Fit Weights Type.ctl" = enum16{"Unweighted", "1/Variance", "Best of All"}
  T64 = typedef "Fits.lvlib/Non-linear Fitting Method v2.ctl" = enum16{"Least Square", "Least Absolute Residual", "Bisquare", "MLE", "-", "Best of All"}
  T65 = typedef "Fits.lvlib/Fit Calculation Method.ctl" = enum16{"Simulation", "Convolution", "Integration"}
  T66 = typedef "Fits.lvlib/Non-linear Fitting Algorithm.ctl" = enum16{"Levenberg-Marquardt", "Trust-Region Dogleg"}
  T67 = typedef "AlliGator Decay Fit.lvlib/AlliGator Decay Fit Parameter Constraints 2.ctl" = cluster{"Fit Parameter":T68, "Min Value":dbl, "Max Value":dbl, "Global":bool, "Used":bool}
  T68 = typedef "Fits.lvlib/Decay Fit Parameters In List.ctl" = enum16{"Offset", "Baseline", "A_1", "tau_1", "A_2", "tau_2"}
  T69 = typedef "Fits.lvlib/MLE Baseline Offset Type.ctl" = enum32{"Absolute", "Percentage"}
  T70 = typedef "AlliGator Decay Preprocessing.lvlib/AlliGator Decay Preprocessing Parameters.ctl" = cluster{"Background Subtraction":bool, "Straighten Decay":bool, "Reverse Gates":bool, "1-Normalized Decay":bool, "Smoothen Decay":bool, "Smoothing Parameter":dbl, "Shift Decay":bool, "Decay Shift Parameters":T50, "Extrapolate Decay":bool, "Additional Points":u32, "Head Fraction":dbl, "Pixel-Normalize Decay":bool, "Use Periodicity":bool, "Use Cursors":bool, "Tail Fraction":dbl, "Use Decay Pre-Processing":bool, "Fold Decay":bool, "# Folds":u32, "[0-1]-Normalized Decay":bool}
  T71 = typedef "Fits.lvlib/Decay Fit Parameters & Derived Quantities List v2.ctl" = enum16{"Offset", "Baseline", "A_1", "tau_1", "A_2", "tau_2", "<tau>_a", "f1_a", "f2_a", "<tau>_i", "f1_i", "f2_i", "-", "R^2", "Chi^2"}
  T72 = typedef "Fits.lvlib/Decay Fit Result Constraint.ctl" = cluster{"Fit Parameter":enum16{"Offset", "Baseline", "A_1", "tau_1", "A_2", "tau_2", "<tau>_a", "f1_a", "f2_a", "<tau>_i", "f1_i", "f2_i", "-", "R^2", "Chi^2", "Max Relative Residual", "<Residual ACF>", "Residual ACF SDV", "tau_2/tau_1"}, "Min Value":dbl, "Max Value":dbl, "Use Constraint":bool}
  T73 = typedef "AlliGator Decay Fit Parameter Map.lvlib/AlliGator Parameter Maps Data.ctl" = cluster{"Map Set Name":string, "[Parameter Names]":string[], "[[Parameters]]":dbl[][], "[[Parameter SDVs]]":dbl[][], "Decay Array Time Axis":dbl[], "[[IRFs]]":dbl[][], "IRF Array Time Axis":dbl[], "X Resolution":i32, "Y Resolution":i32, "Intensity Array":dbl[]}
  T74 = typedef "Phasor.lvlib/Phasor Calibration Type.ctl" = enum16{"None", "Single Phasor", "Phasor Series", "Phasor Map"}
  T75 = cluster{"Use Backup Calibration if needed?":bool, "Calibration Type":T74}
  T76 = cluster{"Selected Plot Info":T17, "Scatter Plot Parameters":T32}
  T77 = typedef "AlliGator Phasor Graph.lvlib/AlliGator Phasor Plot Destination.ctl" = enum32{"Phasor Plot 1", "Phasor Plot 2", "New Phasor Plot"}
  T78 = typedef "AlliGator Phasor Graph.lvlib/AlliGator 2-Phasor Plot Multiplication.ctl" = cluster{"Phasor Plot 1":u16, "Operation 1":T79, "Phasor Plot 2":u16, "Operation 2":T79, "Delay":dbl[unit], "Operation 3":T79, "1-Exp Lifetime":dbl[unit], "Operation 4":T79, "Phasor (g, s)":T22, "Phasor (m, phi)":T36, "Phasor Representation":T80, "Use Operation 1":bool, "Use Operation 2":bool, "Use Operation 3":bool, "Use Operation 4":bool}
  T79 = typedef "Phasor.lvlib/Phasor Operation.ctl" = enum16{"*", "/"}
  T80 = typedef "Phasor.lvlib/Phasor Representation.ctl" = enum32{"(g, s)", "(m, phi)"}
  T81 = typedef "Image.lvlib/Image Save File Format.ctl" = enum16{"PNG", "JPEG", "BMP"}
  T82 = typedef "LVPointDoubleTypeDef.ctl" = cluster{"Cursor X":dbl, "Cursor Y":dbl}
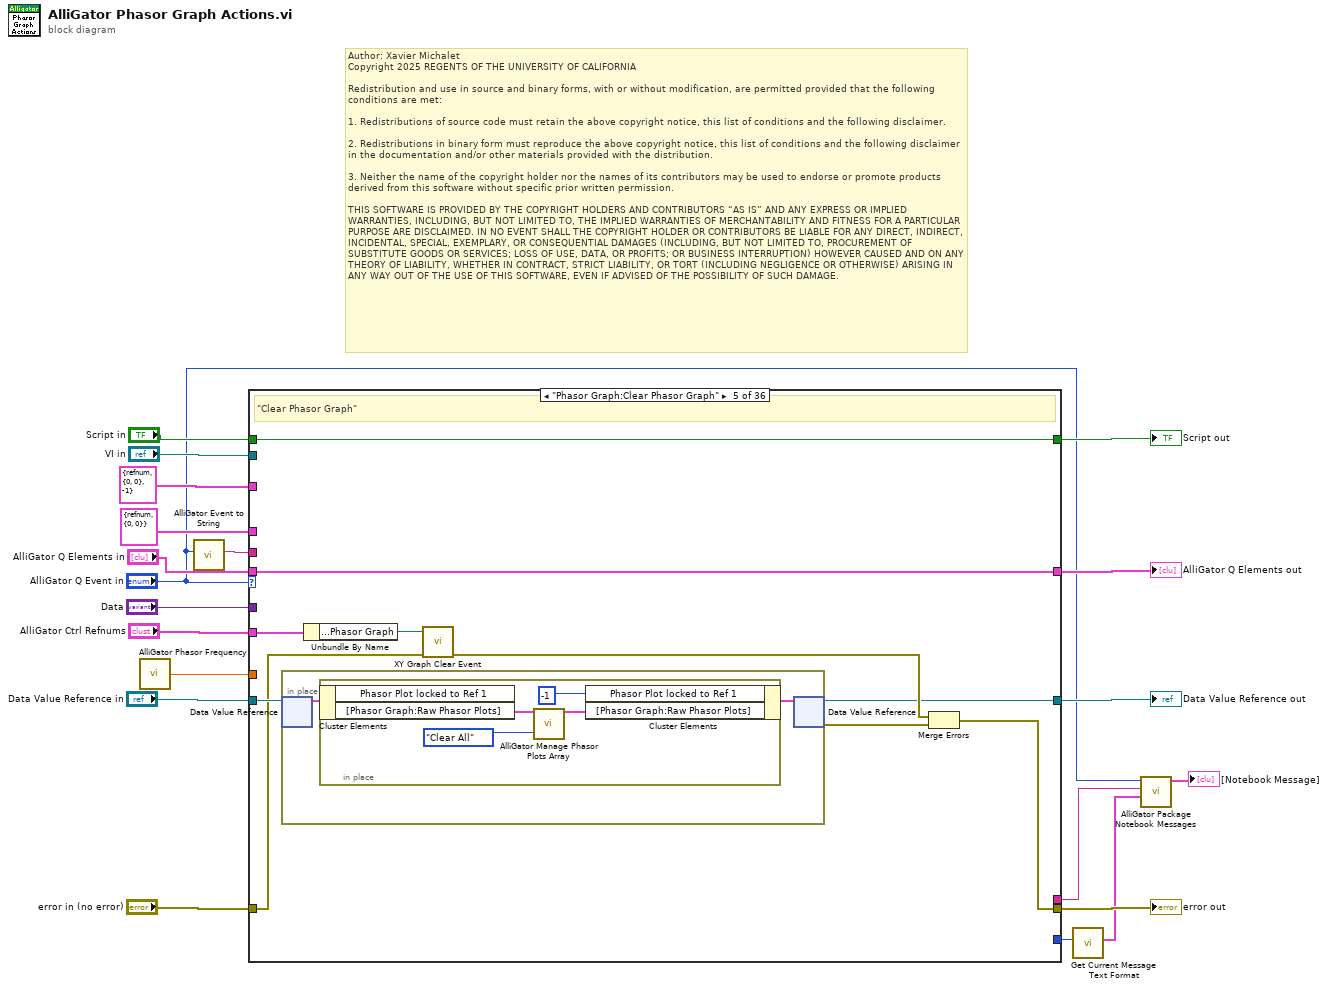
[diagram p0: block diagram]
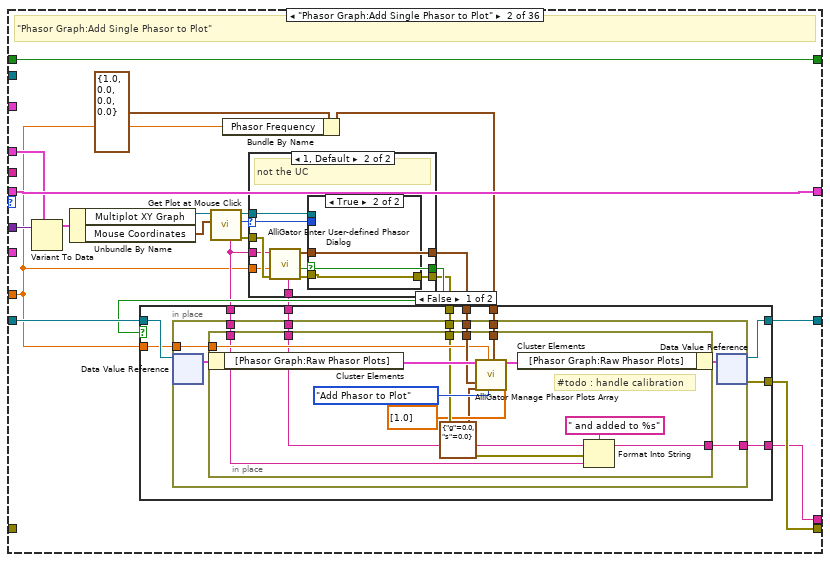
[diagram p3: hidden frame]
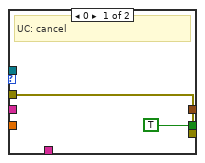
[diagram p4: hidden frame]
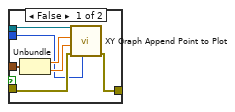
[diagram p5: hidden frame]
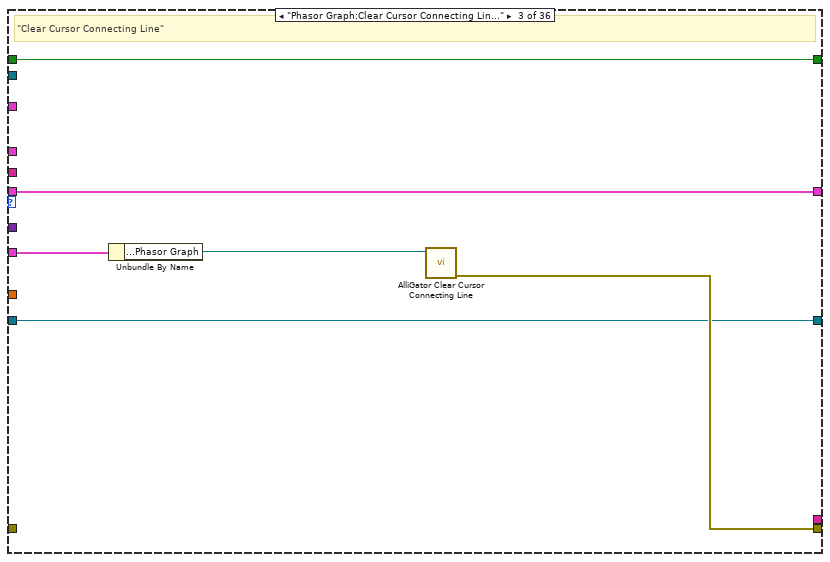
[diagram p7: hidden frame]
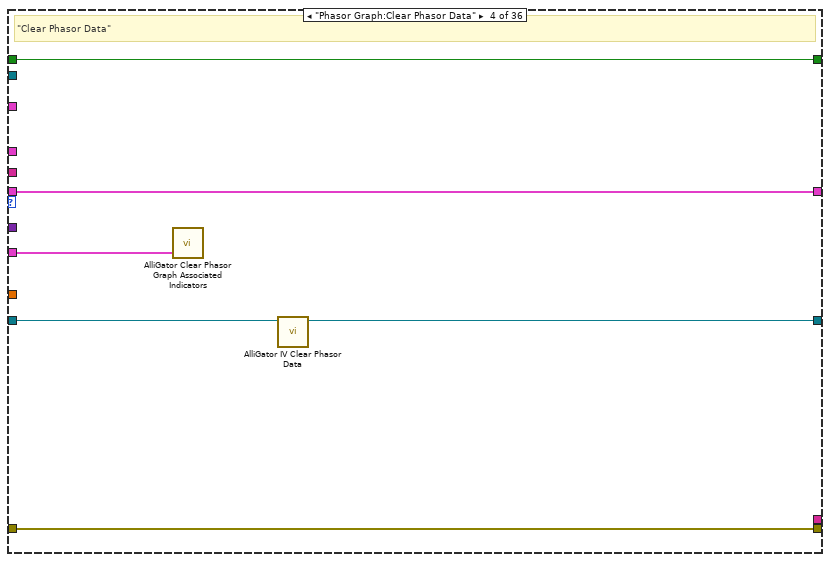
[diagram p8: hidden frame]
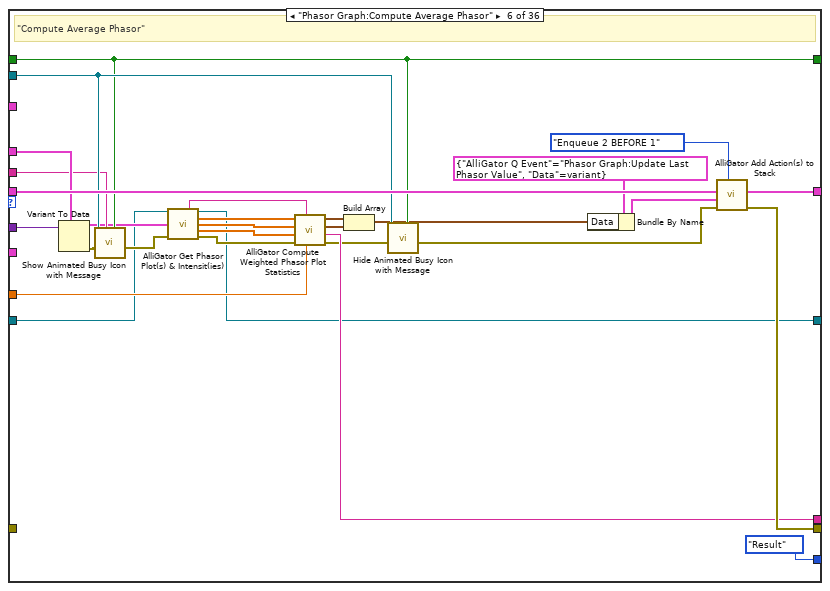
[diagram p9: hidden frame]
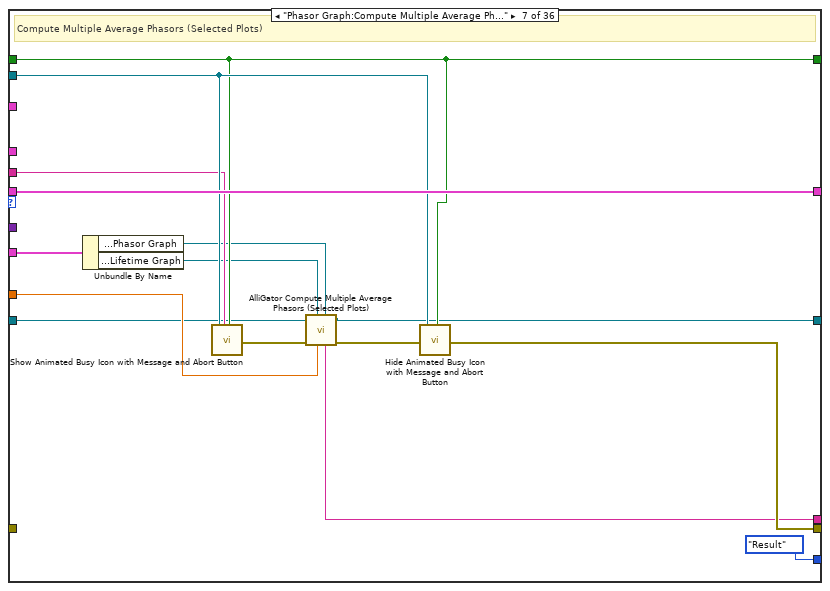
[diagram p10: hidden frame]
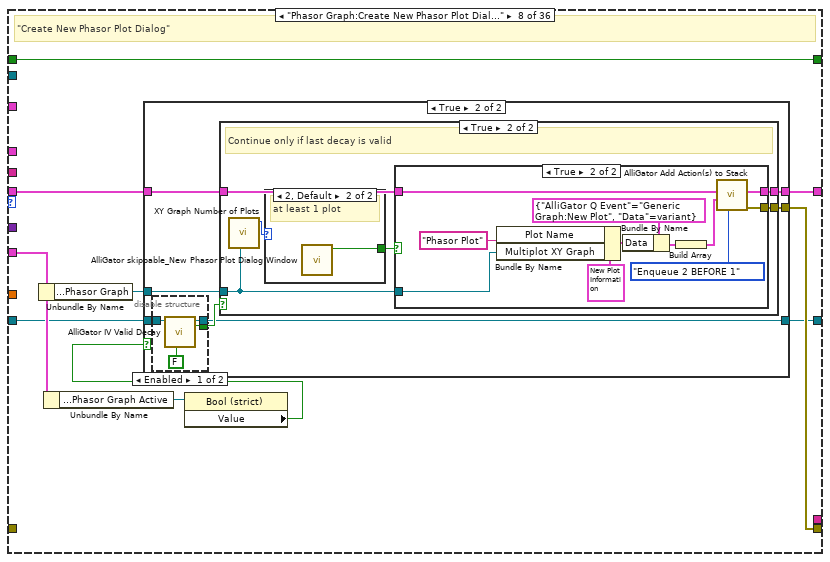
[diagram p11: hidden frame]
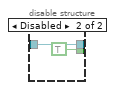
[diagram p13: hidden frame]
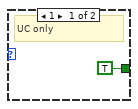
[diagram p15: hidden frame]
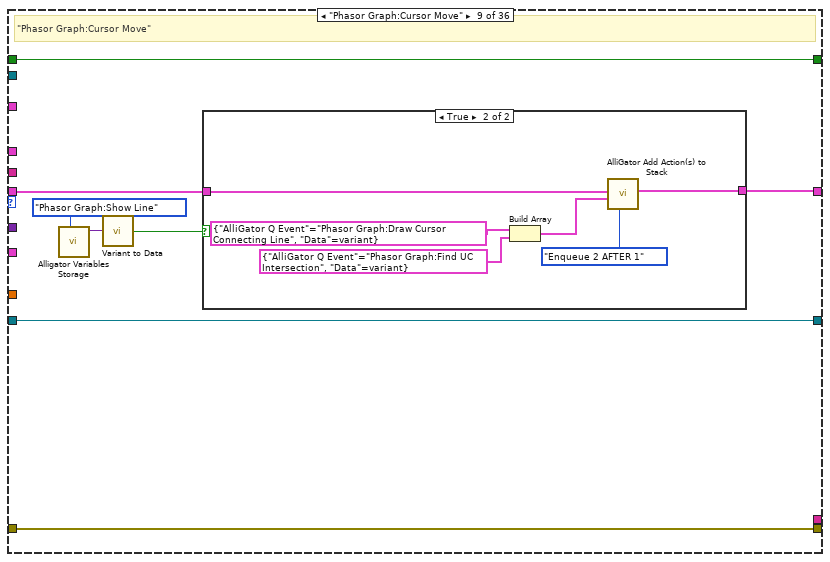
[diagram p17: hidden frame]
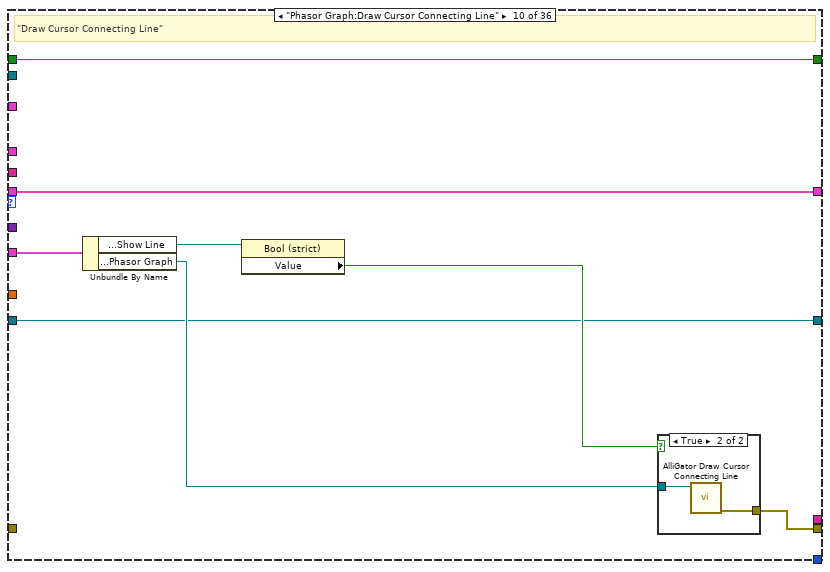
[diagram p19: hidden frame]
diagram:
  # "Author: Xavier Michalet\nCopyright 2025 REGENTS OF THE UNIVERSITY OF CALIFORNIA\n\nRedistribution and use in source and binary forms, with or without modification, are permitted provided that the following conditions are met:\n\n1. Redistributions of source code must retain the above copyright notice, this list of conditions and the following disclaimer.\n\n2. Redistributions in binary form must reproduce the above copyright notice, this list of conditions and the following disclaimer in the documentation and/or other materials provided with the distribution.\n\n3. Neither the name of the copyright holder nor the names of its contributors may be used to endorse or promote products derived from this software without specific prior written permission.\n\nTHIS SOFTWARE IS PROVIDED BY THE COPYRIGHT HOLDERS AND CONTRIBUTORS “AS IS” AND ANY EXPRESS OR IMPLIED WARRANTIES, INCLUDING, BUT NOT LIMITED TO, THE IMPLIED WARRANTIES OF MERCHANTABILITY AND FITNESS FOR A PARTICULAR PURPOSE ARE DISCLAIMED. IN NO EVENT SHALL THE COPYRIGHT HOLDER OR CONTRIBUTORS BE LIABLE FOR ANY DIRECT, INDIRECT, INCIDENTAL, SPECIAL, EXEMPLARY, OR CONSEQUENTIAL DAMAGES (INCLUDING, BUT NOT LIMITED TO, PROCUREMENT OF SUBSTITUTE GOODS OR SERVICES; LOSS OF USE, DATA, OR PROFITS; OR BUSINESS INTERRUPTION) HOWEVER CAUSED AND ON ANY THEORY OF LIABILITY, WHETHER IN CONTRACT, STRICT LIABILITY, OR TORT (INCLUDING NEGLIGENCE OR OTHERWISE) ARISING IN ANY WAY OUT OF THE USE OF THIS SOFTWARE, EVEN IF ADVISED OF THE POSSIBILITY OF SUCH DAMAGE."
  n1 = call "AlliGator Phasor Frequency.vi"() -> ("Phasor Frequency"=w15:dbl[unit])
  n2 = call "AlliGator Event to String.vi"("AlliGator Q Event"="AlliGator Q Event in") -> ("String"=w6:string)  [unwired: 8 in]
  n3 = case shown="\"Phasor Graph:Clear Phasor Graph\"" "AlliGator Q Event in" {
    tunnel: "Data" -> [_ w46 _ _ _ w157 _ _ _ _ w260 w282 w309 _ _ w440 w465 _ _ w511 w522 w537 w572 _ w629 w664 w680 w713 w748 w806 w821 _ w861 w899 w932 _]
    tunnel: "AlliGator Q Elements in" -> [w24 w45 w106 w112 w122 w155 w172 w182 w223 w241 w261 w283 w314 w331 w366 w444 w464 w480 w500 w510 w521 w536 w573 w608 w630 w665 w679 w712 w735 w804 w819 w844 w860 w900 w948 w978]
    tunnel: [w24 w45 w106 w112 w122 w154 w172 w181 w222 w241 w261 w283 w314 w331 w365 w444 w464 w480 w500 w510 w521 w536 w573 w608 w630 w665 w678 w711 w734 w804 w819 w844 w859 w900 w948 w978] -> w11
    tunnel: "VI in" -> [_ _ _ _ _ w147 w168 _ _ _ w246 w264 w302 w317 w357 w437 w447 w469 _ _ _ _ w555 w584 w610 _ _ _ _ _ _ w827 _ w866 w915 w956]
    tunnel: w15 -> [_ w25 _ _ _ w137 w161 _ _ _ _ _ w312 w326 _ _ w452 _ _ _ _ _ _ _ _ _ w675 w706 _ _ _ w835 _ w869 w918 w973]
    tunnel: [w23 w43 w105 w111 w121 w145 w167 w180 w226 w240 w245 w263 w301 w316 w356 w432 w448 w468 w499 w509 w520 w529 w554 w583 w609 w656 w676 w709 w743 w803 w817 w824 w851 w864 w912 w957] -> w12
    tunnel: "Script in" -> [w23 w43 w105 w111 w121 w145 w167 w180 w226 w240 w245 w263 w301 w316 w356 w432 w448 w468 w499 w509 w520 w529 w554 w583 w609 w656 w676 w709 w743 w803 w817 w824 w851 w864 w912 w957]
    tunnel: "error in (no error)" -> [w22 _ _ w107 w113 _ _ _ w225 _ _ _ w305 w324 _ _ w455 _ w498 _ _ _ _ w590 _ _ _ _ _ _ _ w823 _ _ _ w960]
    tunnel: [w22 w32 w103 w107 w115 w148 w169 w178 w225 w238 w247 w281 w303 w323 w364 w434 w449 w476 w498 w504 w515 w528 w556 w586 w619 w655 w674 w705 w742 w791 w809 w830 w850 w871 w922 w958] -> w9
    tunnel: "AlliGator Ctrl Refnums" -> [_ _ w102 w110 w118 _ w165 w176 _ w237 w258 _ w311 w329 w362 w438 w463 w479 _ w502 w513 _ w566 w602 _ w653 w671 _ w740 w801 w815 w829 w848 w876 w927 w966]
    tunnel: "Data Value Reference in" -> [w21 w41 w101 w109 w117 w131 w160 w174 w224 w234 w257 w280 w307 w325 w359 w435 w453 w474 w497 w507 w518 w526 w565 w601 w617 w652 w672 w703 w739 w799 w812 w826 w847 w865 w914 w962]
    tunnel: [w21 w42 w101 w108 w116 w130 w159 w173 w224 w234 w256 w279 w307 w325 w360 w436 w461 w475 w497 w508 w519 w527 w564 w600 w618 w652 w672 w703 w738 w793 w813 w826 w847 w865 w914 w962] -> w20
    tunnel: [_ w29 _ _ _ w140 w164 _ _ _ w249 w265 w306 _ w358 w433 w460 w473 _ w503 w514 w524 w558 w595 w612 w651 w667 w702 _ _ _ _ w845 w863 w913 _] -> w3
    tunnel: T20 {"Multiplot XY Graph"=refnum, "Mouse Coordinates"={"Horizontal"=0, "Vertical"=0}} ("Mouse Click Event Data") -> [_ w40 _ _ _ w146 _ _ _ _ _ _ _ _ _ _ _ _ _ _ _ w525 _ _ _ _ _ _ _ _ _ _ _ _ _ _]
    tunnel: T17 {"Multiplot XY Graph"=refnum, "Mouse Coordinates"={"Horizontal"=0, "Vertical"=0}, "Plot Index"=-1} ("Selected Plot Info") -> [_ _ _ _ _ _ _ _ _ _ _ _ _ _ _ _ _ _ _ _ _ _ _ _ _ _ _ _ _ _ _ _ _ _ _ _]
    tunnel: w6 -> [_ _ _ _ _ w143 w166 _ _ _ w244 w262 w300 w315 w355 w431 w446 w467 _ _ _ _ w553 w585 w611 _ _ _ _ _ _ w822 _ _ _ w955]
    tunnel: [_ _ _ _ _ Text_Format_List."Result" ("Text Format") Text_Format_List."Result" ("Text Format") _ _ _ _ _ _ _ Text_Format_List."Result" ("Text Format") _ Text_Format_List."Result" ("Text Format") Text_Format_List."Result" ("Text Format") _ _ _ _ _ _ _ _ Text_Format_List."Result" ("Text Format") Text_Format_List."Result" ("Text Format") _ _ _ _ _ Text_Format_List."Result" ("Text Format") Text_Format_List."Result" ("Text Format") Text_Format_List."Result" ("Text Format")] -> w1
    frame "---- Phasor Graph ----", Default {
    }
    frame "Phasor Graph:Add Single Phasor to Plot" {
      # "\"Phasor Graph:Add Single Phasor to Plot\""
      n4 = Variant To Data(type=w40, Variant=w46) -> (data=w44:T20)  [unwired: 1 in, 1 out]
      n5 = Unbundle By Name(w44) -> ("Multiplot XY Graph"=w39:T18, "Mouse Coordinates"=w38:T19)
      n6 = call-poly "Get Plot at Mouse Click.vi"("Mouse Click Coordinates"=w38, "XY Graph in"=w39) -> ("error out"=w37:errorcluster, "Plot at Coordinates"=w34:i32, "XY Graph out"=w28:T18, "Plot Name"=w30:string)  [unwired: 3 in, 3 out]
      n7 = Bundle By Name(cluster=T21 {"m"=1.0, "phi"=0.0, "Phasor Frequency"=0.0, "Reference Lifetime"=0.0} ("Calibration Phasor"), "Phasor Frequency"=w25) -> (w26:T21)
      n8 = case shown="1, Default" w34 {
        selector: w34 -> [_ w50]
        tunnel: w37 -> [w47 w58]
        tunnel: w30 -> [_ w57]
        tunnel: w25 -> [_ w56]
        tunnel: [_ w53] -> w36
        tunnel: [TRUE ("Cancelled?") w49] -> w35
        tunnel: [_ w55] -> w33
        tunnel: [w47 w51] -> w31
        tunnel: w28 -> [_ w54]
        frame 0 {
          # "UC: cancel"
        }
        frame 1, Default {
          # "not the UC"
          n9 = call "AlliGator Enter User-defined Phasor Dialog.vi"("Error In"=w58, "Phasor Frequency"=w56, "Phasor Plot Name"=w57) -> ("Error Out"=w52:errorcluster, "Cancelled?"=w49:bool, "New Phasor (g, s)"=w53:T22, "Message"=w55:string)  [unwired: 5 in]
          n10 = case shown="True" w49 {
            tunnel: w54 -> [w65 _]
            tunnel: w53 -> [w64 _]
            tunnel: w52 -> [w61 w66]
            tunnel: [w60 w66] -> w51
            tunnel: w50 -> [w59 _]
            frame False {
              n11 = Unbundle(w64) -> ("g"=w63:dbl, "s"=w62:dbl)
              n12 = call "XY Graph Append Point to Plot.vi"("Plot ID (-1: last)"=w59, "error in (no error)"=w61, "y"=w62, "x"=w63, "XYGraph in"=w65) -> ("error out"=w60:errorcluster)  [unwired: 3 in, 3 out]
            }
            frame True {
            }
          }
        }
      }
      n13 = case shown="False" w35 {
        tunnel: w41 -> [w76 w100]
        tunnel: [w75 w100] -> w42
        tunnel: w36 -> [w74 _]
        tunnel: w33 -> [w70 _]
        tunnel: w25 -> [w73 _]
        tunnel: [w72 w99] -> w32
        tunnel: w31 -> [w71 w99]
        tunnel: w30 -> [w69 _]
        tunnel: [w68 _] -> w29
        tunnel: w26 -> [w67 _]
        frame False {
          n14 = in-place {
            in-place-border: w74 -> [w83]
            in-place-border: w73 -> [w82]
            in-place-border: w71 -> [w81]
            in-place-border: w70 -> [w80]
            in-place-border: w69 -> [w79]
            in-place-border: [w78] -> w68
            in-place-border: w67 -> [w77]
            n15 = in-place-dvr #1(w76) -> (w85:T37)  [unwired: 1 out]
            n16 = in-place {
              in-place-border: w83 -> [w95]
              in-place-border: w82 -> [w94]
              in-place-border: w81 -> [w93]
              in-place-border: w80 -> [w92]
              in-place-border: w79 -> [w90]
              in-place-border: [w89] -> w78
              in-place-border: w77 -> [w88]
              # "#todo : handle calibration"
              n17 = in-place-cluster #2(w85) -> ("[Phasor Graph:Raw Phasor Plots]"=w96:T55[])
              n18 = call "AlliGator Manage Phasor Plots Array.vi"("[Raw Phasor Plot] in"=w96, "Raw Phasor (g, s)"=w95, "Raw Phasor SDV"=T22 {"g"=0.0, "s"=0.0}, "Phasor Frequency"=w94, "[Raw Phasor Plot] Action"=AlliGator_Raw_Phasor_Plot_Array_Action."Add Phasor to Plot", "Calibration Phasor"=w88, "Intensity Array"=dbl[] [1.0]) -> ("[Raw Phasor Plot] out"=w98:T55[])  [unwired: 12 in]
              n19 = in-place-cluster #2("[Phasor Graph:Raw Phasor Plots]"=w98) -> (w84:T37)
              n20 = Format Into String(format string=" and added to %s", initial string=w92, error in=w93, w90) -> (resulting string=w89:string)  [unwired: 1 out]
            }
            n21 = in-place-dvr #1(w84) -> (w75:refnum<data-value>, w72:errorcluster)
          }
        }
        frame True {
        }
      }
    }
    frame "Phasor Graph:Clear Cursor Connecting Line" {
      # "\"Clear Cursor Connecting Line\""
      n22 = Unbundle By Name(w102) -> ("Registered Events Ctrl Refnums.Phasor Graph"=w104:refnum<vi>)
      n23 = call "AlliGator Clear Cursor Connecting Line.vi"("Phasor Graph Refnum"=w104) -> ("Error Out"=w103:errorcluster)  [unwired: 10 in]
    }
    frame "Phasor Graph:Clear Phasor Data" {
      # "\"Clear Phasor Data\""
      n24 = call "AlliGator Clear Phasor Graph Associated Indicators.vi"("AlliGator Ctrl Refnums"=w110) -> ()  [unwired: 11 in]
      n25 = call "AlliGator IV Clear Phasor Data.vi"("Data Value Reference in"=w109) -> ("Data Value Reference out"=w108:refnum<data-value>)  [unwired: 10 in]
    }
    frame "Phasor Graph:Clear Phasor Graph" {
      # "\"Clear Phasor Graph\""
      n26 = in-place {
        n27 = in-place-dvr #3(w117) -> (w124:T37)  [unwired: 1 out]
        n28 = in-place {
          n29 = in-place-cluster #4(w124) -> ("[Phasor Graph:Raw Phasor Plots]"=w128:T55[])  [unwired: 1 out]
          n30 = call "AlliGator Manage Phasor Plots Array.vi"("[Raw Phasor Plot] in"=w128, "[Raw Phasor Plot] Action"=AlliGator_Raw_Phasor_Plot_Array_Action."Clear All") -> ("[Raw Phasor Plot] out"=w127:T55[])  [unwired: 17 in]
          n31 = in-place-cluster #4("Phasor Plot locked to Ref 1"=-1 ("Plot at Coordinates"), "[Phasor Graph:Raw Phasor Plots]"=w127) -> (w123:T37)
        }
        n32 = in-place-dvr #3(w123) -> (w116:refnum<data-value>, w114:errorcluster)
      }
      n33 = Unbundle By Name(w118) -> ("Registered Events Ctrl Refnums.Phasor Graph"=w120:refnum<vi>)
      n34 = call "XY Graph Clear Event.vi"("Error In"=w113, "XYGraph Ref"=w120) -> ("Error Out"=w119:errorcluster)  [unwired: 7 in, 2 out]
      n35 = Merge Errors(w119, w114) -> (w115:errorcluster)
    }
    frame "Phasor Graph:Compute Average Phasor" {
      # "\"Compute Average Phasor\""
      n36 = Variant To Data(type=w146, Variant=w157) -> (data=w132:T20, error out=w156:errorcluster)  [unwired: 1 in]
      n37 = call "Show Animated Busy Icon with Message.vi"("Already active? (F)"=w145, "Message"=w143, "Error In"=w156, "Target VI Refnum"=w147) -> ("Error Out"=w150:errorcluster)  [unwired: 7 in]
      n38 = call "AlliGator Get Phasor Plot(s) & Intensit(ies).vi"("Data Value Reference in"=w131, "Mouse Click Event Data"=w132, "error in (no error)"=w150) -> ("Plot Name(s)"=w133:string, "Data Value Reference out"=w130:refnum<data-value>, "X Array"=w138:dbl[], "Y Array"=w135:dbl[], "Weight Array"=w134:dbl[], "error out"=w136:errorcluster)  [unwired: 7 in]
      n39 = call "AlliGator Compute Weighted Phasor Plot Statistics.vi"("Phasor Frequency"=w137, "Plot Name(s)"=w133, "error in (no error)"=w136, "Intensity Array"=w134, "s Array"=w135, "g Array"=w138) -> ("error out"=w139:errorcluster, "Result String"=w140:string, "Phasor SDV (g, s)"=w141:T22, "Phasor (g, s)"=w142:T22)  [unwired: 2 in]
      n40 = Build Array(w142, w141) -> (w144:T22[])
      n41 = call "Hide Animated Busy Icon with Message.vi"("Already active? (F)"=w145, "Error In"=w139, "Target VI reference"=w147) -> ("Error Out"=w149:errorcluster)  [unwired: 8 in]
      n42 = Bundle By Name(cluster=T6 {"AlliGator Q Event"=enum."Phasor Graph:Update Last Phasor Value", "Data"=variant} ("Alligator Atomic Action"), "Data"=w144) -> (w152:T6)
      n43 = call-poly "AlliGator Add Action(s) to Stack.vi"("Elements Order in Action Stack (Default: 2 BEFORE 1)"=Alligator_Elements_Order_in_Action_Stack."Enqueue 2 BEFORE 1", "Error In"=w149, "Alligator Atomic Action"=w152, "Alligator Queue Element 1"=w155) -> ("Error Out"=w148:errorcluster, "Alligator Queue Element 1 (+ 2)"=w154:T6[])  [unwired: 6 in]
    }
    frame "Phasor Graph:Compute Multiple Average Phasors (Selected Plots)" {
      # "Compute Multiple Average Phasors (Selected Plots)"
      n44 = Unbundle By Name(w165) -> ("Registered Events Ctrl Refnums.Phasor Graph"=w163:refnum<vi>, "Registered Events Ctrl Refnums.Lifetime Graph"=w162:refnum<vi>)
      n45 = call "Show Animated Busy Icon with Message and Abort Button.vi"("Already active? (F)"=w167, "Message"=w166, "Target VI reference"=w168) -> ("Error Out"=w170:errorcluster)  [unwired: 16 in]
      n46 = call "AlliGator Compute Multiple Average Phasors (Selected Plots).vi"("Phasor Graph Ref"=w163, "Phasor Frequency"=w161, "Lifetime Graph Ref"=w162, "error in (no error)"=w170, "Data Value Reference in"=w160) -> ("error out"=w171:errorcluster, "Data Value Reference out"=w159:refnum<data-value>, "Result String"=w164:string)  [unwired: 2 in, 2 out]
      n47 = call "Hide Animated Busy Icon with Message and Abort Button.vi"("Already active? (F)"=w167, "Target VI reference"=w168, "Error In"=w171) -> ("Error Out"=w169:errorcluster)  [unwired: 16 in]
    }
    frame "Phasor Graph:Create New Phasor Plot Dialog" {
      # "\"Create New Phasor Plot Dialog\""
      n48 = Unbundle By Name(w176) -> ("Registered Events Ctrl Refnums.Phasor Graph"=w179:refnum<vi>)
      n49 = Unbundle By Name(w176) -> ("Phasor Graph Ctrl Refnums.Phasor Graph Active"=w177:refnum<vi>)
      n50 = property class="Bool (strict)"(reference=w177) -> ("Value"=w175:bool)  [unwired: 1 in, 2 out]
      n51 = case shown="True" w175 {
        tunnel: w182 -> [w184 w191]
        tunnel: [w184 w190] -> w181
        tunnel: w179 -> [_ w189]
        tunnel: [_ w188] -> w178
        tunnel: w174 -> [w183 w187]
        tunnel: [w183 w185] -> w173
        frame False {
        }
        frame True {
          n52 = disable-structure shown="Enabled" {
            disable-tunnel: w187 -> [w195 w197]
            disable-tunnel: [w193 TRUE ("Valid Decay")] -> w186
            disable-tunnel: [w192 w197] -> w185
            frame Enabled {
              n53 = call "AlliGator IV Valid Decay.vi"("Get (F)/ Set (T)"=FALSE, "AlliGator IV DVR in"=w195) -> ("Valid Decay"=w193:bool, "AlliGator IV DVR out"=w192:refnum<data-value>)  [unwired: 7 in, 1 out]
            }
            frame Disabled {
            }
          }
          n54 = case shown="True" w186 {
            tunnel: w191 -> [w198 w204]
            tunnel: [w198 w203] -> w190
            tunnel: w189 -> [_ w200]
            tunnel: [_ w199] -> w188
            frame False {
              # "Last decay invalid"
            }
            frame True {
              # "Continue only if last decay is valid"
              n55 = call "XY Graph Number of Plots.vi"("XYGraph in"=w200) -> ("# Plots"=w201:i32)  [unwired: 9 in, 1 out]
              n56 = case shown="2, Default" w201 {
                tunnel: [TRUE ("T button?") w206] -> w202
                frame 1 {
                  # "UC only"
                }
                frame 2, Default {
                  # "at least 1 plot"
                  n57 = call "AlliGator skippable_New Phasor Plot Dialog Window.vi"() -> ("New Plot?"=w206:bool)  [unwired: 10 in, 1 out]
                }
              }
              n58 = case shown="True" w202 {
                tunnel: w204 -> [w207 w218]
                tunnel: [w207 w217] -> w203
                tunnel: w200 -> [_ w213]
                tunnel: [_ w212] -> w199
                frame False {
                }
                frame True {
                  n59 = Bundle By Name(cluster=T26 {"Multiplot XY Graph"=refnum, "Plot Name"="", "Plot Scales"={"X Scale"=0, "Y Scale"=0}, "Plot Interpolation"=enum."Point (.)", "Point Style"=enum."Empty Square", "Plot Color"=15781887, "Plot Metadata"=variant} ("New Plot Information"), "Plot Name"="Phasor Plot", "Multiplot XY Graph"=w213) -> (w211:T26)
                  n60 = Bundle By Name(cluster=T6 {"AlliGator Q Event"=enum."Generic Graph:New Plot", "Data"=variant} ("Alligator Atomic Action"), "Data"=w211) -> (w209:T6)
                  n61 = Build Array(w209) -> (w215:T6[])
                  n62 = call-poly "AlliGator Add Action(s) to Stack.vi"("Elements Order in Action Stack (Default: 2 BEFORE 1)"=Alligator_Elements_Order_in_Action_Stack."Enqueue 2 BEFORE 1", "Alligator Queue Element 2"=w215, "Alligator Queue Element 1"=w218) -> ("Error Out"=w212:errorcluster, "Alligator Queue Element 1 (+ 2)"=w217:T6[])  [unwired: 7 in]
                }
              }
            }
          }
        }
      }
    }
    frame "Phasor Graph:Cursor Move" {
      # "\"Phasor Graph:Cursor Move\""
      n63 = call "Alligator Variables Storage.vi"("AlliGator Variable"=AlliGator_Variables_List."Phasor Graph:Show Line") -> ("Data out"=w220:variant)  [unwired: 8 in, 2 out]
      n64 = call-poly "Variant to Data.vi"("Variant"=w220) -> ("Value"=w219:bool)  [unwired: 8 in]
      n65 = case shown="True" w219 {
        tunnel: w223 -> [w227 w231]
        tunnel: [w227 w229] -> w222
        frame False {
        }
        frame True {
          n66 = Build Array(T6 {"AlliGator Q Event"=enum."Phasor Graph:Draw Cursor Connecting Line", "Data"=variant} ("Time-Gated Phasor Q Element"), T6 {"AlliGator Q Event"=enum."Phasor Graph:Find UC Intersection", "Data"=variant} ("Time-Gated Phasor Q Element")) -> (w230:T6[])
          n67 = call-poly "AlliGator Add Action(s) to Stack.vi"("Elements Order in Action Stack (Default: 2 BEFORE 1)"=Alligator_Elements_Order_in_Action_Stack."Enqueue 2 AFTER 1", "Alligator Queue Element 2"=w230, "Alligator Queue Element 1"=w231) -> ("Alligator Queue Element 1 (+ 2)"=w229:T6[])  [unwired: 7 in, 1 out]
        }
      }
    }
    frame "Phasor Graph:Draw Cursor Connecting Line" {
      # "\"Draw Cursor Connecting Line\""
      n68 = Unbundle By Name(w237) -> ("Phasor Graph Ctrl Refnums.Show Line"=w236:refnum<vi>, "Registered Events Ctrl Refnums.Phasor Graph"=w239:refnum<vi>)
      n69 = property class="Bool (strict)"(reference=w236) -> ("Value"=w235:bool)  [unwired: 1 in, 2 out]
      n70 = case shown="True" w235 {
        tunnel: w239 -> [_ w243]
        tunnel: [_ w242] -> w238
        frame False {
        }
        frame True {
          n71 = call "AlliGator Draw Cursor Connecting Line.vi"("Phasor Graph Refnum"=w243) -> ("Error Out"=w242:errorcluster)  [unwired: 10 in]
        }
      }
    }
    frame "Phasor Graph:Export Selected Phasor Plots Data" {
      w254 = TRUE  # Save as...
      # "\"Export Selected Phasor Plots Data\""
      n72 = call-poly "Variant to Data.vi"("Variant"=w260) -> ("Value"=w253:bool)  [unwired: 8 in]
      n73 = Unbundle By Name(w258) -> ("Registered Events Ctrl Refnums.Phasor Graph"=w255:refnum<vi>)
      n74 = call "AlliGator IV [Raw Phasor Plot].vi"("Get (F)/ Set (T)"=FALSE, "AlliGator IV DVR in"=w257) -> ("error out"=w251:errorcluster, "[Raw Phasor Plots]"=w252:T55[], "AlliGator IV DVR out"=w256:refnum<data-value>)  [unwired: 7 in]
      n75 = call "Show Animated Busy Icon with Message.vi"("Already active? (F)"=w245, "Message"=w244, "Error In"=w251, "Target VI Refnum"=w246) -> ("Error Out"=w248:errorcluster)  [unwired: 7 in]
      n76 = call "AlliGator Save Multiple Phasor Plots Additional Data.vi"("Save as..."=w254, "error in (no error)"=w248, "Raw Phasor Plots"=w252, "All Plots"=w253, "Phasor Graph"=w255) -> ("Error Out"=w259:errorcluster, "Message"=w249:string)  [unwired: 5 in]
      n77 = call "Hide Animated Busy Icon with Message.vi"("Already active? (F)"=w245, "Error In"=w259, "Target VI reference"=w246) -> ("Error Out"=w247:errorcluster)  [unwired: 8 in]
    }
    frame "Phasor Graph:Export Single Phasor Plot Data" {
      # "\"Export Single Phasor Plot Data\""
      n78 = Variant To Data(type=T31 {"Mouse Click Event Data"={"Multiplot XY Graph"=refnum, "Mouse Coordinates"={"Horizontal"=0, "Vertical"=0}}, "Save as..."=FALSE} ("output cluster"), Variant=w282) -> (data=w278:T31, error out=w267:errorcluster)  [unwired: 1 in]
      n79 = Unbundle(w278) -> ("Mouse Click Event Data"=w277:T20, "Save as..."=w271:bool)
      n80 = call "AlliGator IV [Raw Phasor Plot].vi"("Get (F)/ Set (T)"=FALSE, "error in (no error)"=w267, "AlliGator IV DVR in"=w280) -> ("error out"=w266:errorcluster, "[Raw Phasor Plots]"=w269:T55[], "AlliGator IV DVR out"=w279:refnum<data-value>)  [unwired: 6 in]
      n81 = Unbundle(w277) -> ("Multiplot XY Graph"=w273:T18, "Mouse Coordinates"=w272:T19)
      n82 = call-poly "Get Plot at Mouse Click.vi"("error in (no error)"=w266, "Mouse Click Coordinates"=w272, "XY Graph in"=w273) -> ("error out"=w276:errorcluster, "Plot at Coordinates"=w270:i32, "XY Graph out"=w275:T18)  [unwired: 2 in, 4 out]
      n83 = case shown="1, Default" w270 {
        selector: w270 -> [_ w293]
        tunnel: w276 -> [w284 w298]
        tunnel: w275 -> [_ w299]
        tunnel: w271 -> [_ w297]
        tunnel: w269 -> [_ w295]
        tunnel: [w284 w288] -> w281
        tunnel: [_ w290] -> w265
        tunnel: w264 -> [_ w287]
        tunnel: w263 -> [_ w286]
        tunnel: w262 -> [_ w285]
        frame -1, 0 {
          # "UC or not found"
        }
        frame 1, Default {
          n84 = Decrement(x=w293) -> (x-1=w296:i32)
          n85 = call "Show Animated Busy Icon with Message.vi"("Already active? (F)"=w286, "Message"=w285, "Error In"=w298, "Target VI Refnum"=w287) -> ("Error Out"=w289:errorcluster)  [unwired: 7 in]
          n86 = Index Array(array=w295, index=w296) -> (element=w294:T55)
          n87 = call "AlliGator Script Destination File Path.vi"() -> ("Destination File Path"=w292:path)
          n88 = call "AlliGator Save Phasor Plot Additional Data.vi"("Save as..."=w297, "Phasor Plot Folder Path (empty)"=w292, "error in (no error)"=w289, "Raw Phasor Plot"=w294, "Selected Plot"=w293, "Phasor Graph"=w299) -> ("Error Out"=w291:errorcluster, "Message"=w290:string)  [unwired: 4 in]
          n89 = call "Hide Animated Busy Icon with Message.vi"("Already active? (F)"=w286, "Error In"=w291, "Target VI reference"=w287) -> ("Error Out"=w288:errorcluster)  [unwired: 8 in]
        }
      }
    }
    frame "Phasor Graph:Export Single Phasor Plot Phase Lifetimes" {
      # "\"Export Single Phasor Plot Phase Lifetime\""
      n90 = Unbundle By Name(w311) -> ("Registered Events Ctrl Refnums.Phasor Graph"=w310:refnum<vi>)
      n91 = call-poly "Variant to Data.vi"("Variant"=w309) -> ("Path"=w308:path)  [unwired: 8 in]
      n92 = call "Show Animated Busy Icon with Message.vi"("Already active? (F)"=w301, "Message"=w300, "Error In"=w305, "Target VI Refnum"=w302) -> ("Error Out"=w304:errorcluster)  [unwired: 7 in]
      n93 = call "AlliGator Export Single Phasor Plot Phase Lifetimes.vi"("Frequency"=w312, "Error In"=w304, "File Path in (empty: dialog)"=w308, "Phasor Graph"=w310) -> ("Error Out"=w313:errorcluster, "Message"=w306:string)  [unwired: 5 in, 1 out]
      n94 = call "Hide Animated Busy Icon with Message.vi"("Already active? (F)"=w301, "Error In"=w313, "Target VI reference"=w302) -> ("Error Out"=w303:errorcluster)  [unwired: 8 in]
    }
    frame "Phasor Graph:Find UC Intersection" {
      # "\"Find UC Intersection\""
      n95 = Unbundle By Name(w329) -> ("Phasor Graph Ctrl Refnums.Phasor Reference 1 Control"=w320:refnum<vi>, "Phasor Graph Ctrl Refnums.Phasor Reference 2 Control"=w319:refnum<vi>, "Registered Events Ctrl Refnums.Phasor Graph"=w330:refnum<vi>, "Phasor Graph Ctrl Refnums.Phase Lifetime 1"=w328:refnum<vi>, "Phasor Graph Ctrl Refnums.Phase Lifetime 2"=w327:refnum<vi>)
      n96 = property class="Scroll (strict)"(reference=w320) -> ("Visible"=w322:bool)  [unwired: 1 in, 2 out]
      n97 = property class="Scroll (strict)"(reference=w319) -> ("Visible"=w321:bool)  [unwired: 1 in, 2 out]
      n98 = Or(x=w322, y=w321) -> (x .or. y?=w318:bool)
      n99 = case shown="True" w318 {
        tunnel: w330 -> [_ w352]
        tunnel: w328 -> [_ w351]
        tunnel: w327 -> [_ w350]
        tunnel: w326 -> [_ w347]
        tunnel: w324 -> [w332 w344]
        tunnel: [w332 w336] -> w323
        tunnel: w317 -> [_ w334]
        tunnel: w316 -> [_ w333]
        tunnel: w315 -> [_ w335]
        frame False {
        }
        frame True {
          w345 = TRUE ("Visible")
          n100 = call "Show Animated Busy Icon with Message.vi"("Already active? (F)"=w333, "Message"=w335, "Error In"=w344, "Target VI Refnum"=w334) -> ("Error Out"=w337:errorcluster)  [unwired: 7 in]
          n101 = call "AlliGator Find Cursor Connecting Line Intersection(s) with Universal Circle.vi"("Error In"=w337, "XY Graph Refnum"=w352) -> ("Error Out"=w342:errorcluster, "Intersection 2"=w348:cluster{"x":dbl, "y":dbl}, "Intersection 1"=w353:cluster{"x":dbl, "y":dbl})  [unwired: 7 in]
          n102 = call "Phasor Convert (g,s,f) to (tf, tm).vi"("Error In"=w342, "Phasor Harmonic Frequency"=w347, "Phasor (g, s)"=w353) -> ("Error Out"=w343:errorcluster, "Phase Lifetime"=w349:dbl[unit])  [unwired: 6 in, 1 out]
          n103 = call "Phasor Convert (g,s,f) to (tf, tm).vi"("Error In"=w342, "Phasor Harmonic Frequency"=w347, "Phasor (g, s)"=w348) -> ("Error Out"=w341:errorcluster, "Phase Lifetime"=w346:dbl[unit])  [unwired: 6 in, 1 out]
          n104 = property class="DigNum (strict)"(reference=w351, error in=w343, "Value"=w349, "Visible"=w345) -> (error out=w340:errorcluster)  [unwired: 1 out]
          n105 = property class="DigNum (strict)"(reference=w350, error in=w341, "Value"=w346, "Visible"=w345) -> (error out=w339:errorcluster)  [unwired: 1 out]
          n106 = Merge Errors(w340, w339) -> (w338:errorcluster)
          n107 = call "Hide Animated Busy Icon with Message.vi"("Already active? (F)"=w333, "Error In"=w338, "Target VI reference"=w334) -> ("Error Out"=w336:errorcluster)  [unwired: 8 in]
        }
      }
    }
    frame "Phasor Graph:Get Phasor Value" {
      # "\"Get Phasor Value\""
      n108 = Unbundle By Name(w362) -> ("Phasor Graph Ctrl Refnums.Phasor Graph Active"=w363:refnum<vi>)
      n109 = property class="Bool (strict)"(reference=w363) -> ("Value"=w361:bool)  [unwired: 1 in, 2 out]
      n110 = case shown="True" w361 {
        tunnel: w366 -> [w368 w384]
        tunnel: [w368 w383] -> w365
        tunnel: [_ w377] -> w364
        tunnel: w362 -> [_ w379]
        tunnel: [w367 w378] -> w360
        tunnel: w359 -> [w367 w376]
        tunnel: [_ w372] -> w358
        tunnel: w357 -> [_ w371]
        tunnel: w356 -> [_ w370]
        tunnel: w355 -> [_ w369]
        frame False {
        }
        frame True {
          n111 = Unbundle By Name(w379) -> ("Phasor Graph Ctrl Refnums.Save Phasor Graph"=w381:refnum<vi>, "Registered Events Ctrl Refnums.Phasor Graph"=w382:refnum<vi>, "Phasor Graph Ctrl Refnums.Single Step Phasor"=w374:refnum<vi>, "Phasor Graph Ctrl Refnums.Phasor Frame Slide"=w380:refnum<vi>)
          n112 = disable-structure shown="Enabled" {
            disable-tunnel: w376 -> [w388 w390]
            disable-tunnel: [w387 w390] -> w375
            disable-tunnel: [w385 TRUE ("Valid Decay")] -> w373
            frame Enabled {
              n113 = call "AlliGator IV Valid Decay.vi"("Get (F)/ Set (T)"=FALSE, "AlliGator IV DVR in"=w388) -> ("Valid Decay"=w385:bool, "AlliGator IV DVR out"=w387:refnum<data-value>)  [unwired: 7 in, 1 out]
            }
            frame Disabled {
            }
          }
          n114 = case shown="True" w373 {
            tunnel: w384 -> [w392 w425]
            tunnel: [w392 w424] -> w383
            tunnel: w382 -> [_ w405]
            tunnel: w381 -> [_ w419]
            tunnel: w380 -> [_ w417]
            tunnel: [w391 w406] -> w378
            tunnel: [_ w411] -> w377
            tunnel: w375 -> [w391 w408]
            tunnel: w374 -> [_ w404]
            tunnel: [_ w402] -> w372
            tunnel: w371 -> [_ w398]
            tunnel: w370 -> [_ w397]
            tunnel: w369 -> [_ w396]
            frame False {
            }
            frame True {
              n115 = call "AlliGator IV Dataset Path.vi"("Get (F)/ Set (T)"=FALSE, "AlliGator IV DVR in"=w408) -> ("error out"=w414:errorcluster, "AlliGator IV DVR out"=w407:refnum<data-value>, "Current Dataset"=w413:i32)  [unwired: 5 in, 2 out]
              n116 = property class="Bool (strict)"(reference=w419) -> ("Value"=w418:bool)  [unwired: 1 in, 2 out]
              n117 = Increment(x=w413) -> (x+1=w416:i32)
              n118 = call "Show Animated Busy Icon with Message.vi"("Already active? (F)"=w397, "Message"=w396, "Error In"=w414, "Target VI Refnum"=w398) -> ("Error Out"=w395:errorcluster)  [unwired: 7 in]
              n119 = call "AlliGator Get Basic Calibration Options.vi"("error in (no error)"=w395) -> ("error out"=w394:errorcluster, "Basic Calibration Options"=w393:T75)  [unwired: 9 in]
              n120 = call "AlliGator Get Phasor Value from Decay.vi"("Basic Calibration Options"=w393, "Error In"=w394, "Single Step Phasor"=w404, "Phasor Graph in"=w405, "AlliGator Internal Variables DVR"=w407) -> ("Error Out"=w410:errorcluster, "Calibrated Phasor SDV"=w400:T22, "Calibrated Phasor"=w403:T22, "AlliGator Internal Variables DVR"=w406:refnum<data-value>, "Message"=w402:string)  [unwired: 1 in, 1 out]
              n121 = Build Array(w403, w400) -> (w401:T22[])
              n122 = property class="Slide (strict)"(reference=w417, error in=w410, "Scale.Maximum"=w416, "Scale.Minimum"=1.0 ("Scale.Range:Maximum"), "Value"=w416) -> (error out=w409:errorcluster)  [unwired: 1 out]
              n123 = Bundle By Name(cluster=T6 {"AlliGator Q Event"=enum."Phasor Graph:Update Last Phasor Value", "Data"=variant} ("Alligator Atomic Action"), "Data"=w401) -> (w421:T6)
              n124 = case shown="True" w418 {
                tunnel: w421 -> [w427 w429]
                tunnel: [w426 w430] -> w420
                frame False {
                  n125 = Build Array(w427) -> (w426:T6[])
                }
                frame True {
                  n126 = Build Array(T6 {"AlliGator Q Event"=enum."Phasor Graph:Save Phasor Graph Image", "Data"=variant} ("element"), w429) -> (w430:T6[])
                }
              }
              n127 = call "Hide Animated Busy Icon with Message.vi"("Already active? (F)"=w397, "Error In"=w409, "Target VI reference"=w398) -> ("Error Out"=w399:errorcluster)  [unwired: 8 in]
              n128 = call-poly "AlliGator Add Action(s) to Stack.vi"("Elements Order in Action Stack (Default: 2 BEFORE 1)"=Alligator_Elements_Order_in_Action_Stack."Enqueue 2 BEFORE 1", "Error In"=w399, "Alligator Queue Element 2"=w420, "Alligator Queue Element 1"=w425) -> ("Error Out"=w411:errorcluster, "Alligator Queue Element 1 (+ 2)"=w424:T6[])  [unwired: 6 in]
            }
          }
        }
      }
    }
    frame "Phasor Graph:Load Phasor Plot(s)" {
      # "\"Load Phasor Plot(s)\""
      n129 = Unbundle By Name(w438) -> ("Registered Events Ctrl Refnums.Phasor Graph"=w443:refnum<vi>)
      n130 = call-poly "Variant to Data.vi"("Variant"=w440) -> ("Value"=w439:path[])  [unwired: 8 in]
      n131 = call "Show Animated Busy Icon with Message.vi"("Already active? (F)"=w432, "Message"=w431, "Target VI Refnum"=w437) -> ("Error Out"=w442:errorcluster)  [unwired: 8 in]
      n132 = call "AlliGator Load Phasor Plot(s).vi"("Phasor Graph refnum"=w443, "error in (no error)"=w442, "File paths"=w439, "AlliGator IV DVR"=w435) -> ("error out"=w441:errorcluster, "Message"=w433:string, "AlliGator IV DVR"=w436:refnum<data-value>)  [unwired: 5 in]
      n133 = call "Hide Animated Busy Icon with Message.vi"("Already active? (F)"=w432, "Error In"=w441, "Target VI reference"=w437) -> ("Error Out"=w434:errorcluster)  [unwired: 8 in]
    }
    frame "Phasor Graph:Parameter 2 vs Parameter 1 Scatter Plot" {
      # "\"Phasor Graph:Parameter 2 vs Parameter 1 Scatter Plot\""
      n134 = Unbundle By Name(w463) -> ("Registered Events Ctrl Refnums.Lifetime Graph"=w451:refnum<vi>)
      n135 = Bundle("Selected Plot Info"=T17 {"Multiplot XY Graph"=refnum, "Mouse Coordinates"={"Horizontal"=0, "Vertical"=0}, "Plot Index"=-1}, "Scatter Plot Parameters"=T32 {"Parameter 2"=enum."Phasor g", "Parameter 1"=enum."Phasor g"}) -> (w457:T76)  [unwired: 1 in]
      n136 = Variant To Data(error in=w455, type=w457, Variant=w465) -> (data=w454:T76, error out=w462:errorcluster)
      n137 = call "Show Animated Busy Icon with Message.vi"("Already active? (F)"=w448, "Message"=w446, "Error In"=w462, "Target VI Refnum"=w447) -> ("Error Out"=w450:errorcluster)  [unwired: 7 in]
      n138 = call "AlliGator Compute P2 vs P1 Plots.vi"("Lifetime Graph in"=w451, "error in (no error)"=w450, "Phasor Frequency"=w452, "User Selection"=w454, "AlliGator IV DVR in"=w453) -> ("error out"=w459:errorcluster, "Message"=w460:string, "AlliGator IV DVR out"=w461:refnum<data-value>)  [unwired: 4 in]
      n139 = call "Hide Animated Busy Icon with Message.vi"("Already active? (F)"=w448, "Error In"=w459, "Target VI reference"=w447) -> ("Error Out"=w449:errorcluster)  [unwired: 8 in]
    }
    frame "Phasor Graph:Phasor Multiplication" {
      # "\"Phasor Graph:Phasor Algebra\""
      n140 = Unbundle By Name(w479) -> ("Registered Events Ctrl Refnums.Phasor Graph"=w471:refnum<vi>)
      n141 = call "AlliGator Phasor Plot Multiplication Window.vi"("Phasor Graph"=w471) -> ("Error Out"=w477:errorcluster, "Cancelled"=w472:bool, "Phasor Plot Destination Output"=w470:T77, "Phasor Plot Algebra Output"=w478:T78)  [unwired: 7 in]
      n142 = case shown="False" w472 {
        tunnel: w478 -> [w487 _]
        tunnel: w477 -> [w493 w494]
        tunnel: [w484 w494] -> w476
        tunnel: [w491 w495] -> w475
        tunnel: w474 -> [w490 w495]
        tunnel: [w489 _] -> w473
        tunnel: w471 -> [w488 _]
        tunnel: w470 -> [w486 _]
        tunnel: w469 -> [w482 _]
        tunnel: w468 -> [w481 _]
        tunnel: w467 -> [w483 _]
        frame False {
          n143 = call "Show Animated Busy Icon with Message.vi"("Already active? (F)"=w481, "Message"=w483, "Error In"=w493, "Target VI Refnum"=w482) -> ("Error Out"=w485:errorcluster)  [unwired: 7 in]
          n144 = call "AlliGator Phasor Algebra Calculator.vi"("XYGraph in"=w488, "error in (no error)"=w485, "Phasor Plot Destination"=w486, "Phasor Plot Algebra Output"=w487, "Data Value Reference in"=w490) -> ("error out"=w492:errorcluster, "Message"=w489:string, "Data Value Reference out"=w491:refnum<data-value>)  [unwired: 4 in]
          n145 = call "Hide Animated Busy Icon with Message.vi"("Already active? (F)"=w481, "Error In"=w492, "Target VI reference"=w482) -> ("Error Out"=w484:errorcluster)  [unwired: 8 in]
        }
        frame True {
        }
      }
    }
    frame "Phasor Graph:Python Function Phasor Graph Event" {
      # "\"Phasor Graph:Python Function Phasor Graph Event\""
      n146 = One Button Dialog(message="Not yet supported....") -> ()  [unwired: 1 in, 1 out]
      n147 = call "Play Error Sound.vi"() -> ()  [unwired: 27 in, 1 out]
    }
    frame "Phasor Graph:Remove Phasor Plot" {
      # "\"Phasor Graph:Remove Phasor Plot\""
      n148 = Variant To Data(Variant=w511) -> (data=w506:T17, error out=w505:errorcluster)  [unwired: 2 in]
      n149 = Unbundle By Name(w502) -> ("Phasor Graph Ctrl Refnums.Phasor Reference 1 Control"=w501:refnum<vi>)
      n150 = call "AlliGator Remove Phasor Plot.vi"("error in (no error)"=w505, "Phasor Reference 1 Refnum"=w501, "Selected Plot Info"=w506, "AlliGator IV DVR in"=w507) -> ("error out"=w504:errorcluster, "Message"=w503:string, "AlliGator IV DVR out"=w508:refnum<data-value>)  [unwired: 5 in]
    }
    frame "Phasor Graph:Remove Selected Phasor Plots" {
      # "\"Phasor Graph:Remove Selected Phasor Plots\""
      n151 = Variant To Data(Variant=w522) -> (data=w517:T17, error out=w516:errorcluster)  [unwired: 2 in]
      n152 = Unbundle By Name(w513) -> ("Phasor Graph Ctrl Refnums.Phasor Reference 1 Control"=w512:refnum<vi>)
      n153 = call "AlliGator Remove Selected Phasor Plots.vi"("error in (no error)"=w516, "Phasor Reference 1 Refnum"=w512, "Selected Plot Info"=w517, "AlliGator IV DVR in"=w518) -> ("error out"=w515:errorcluster, "Message"=w514:string, "AlliGator IV DVR out"=w519:refnum<data-value>)  [unwired: 5 in]
    }
    frame "Phasor Graph:Remove Single Phasor from Plot" {
      w523 = i32[] [0]  # Excludes UC
      # "Remove Single Phasor from Plot"
      n154 = Variant To Data(type=w525, Variant=w537) -> (data=w535:T20)  [unwired: 1 in, 1 out]
      n155 = Unbundle By Name(w535) -> ("Multiplot XY Graph"=w533:T18, "Mouse Coordinates"=w534:T19)
      n156 = call "XY Graph Remove Data Point.vi"("Excluded Plots"=w523, "Coords"=w534, "XYGraph in"=w533) -> ("Error Out"=w528:errorcluster, "Point  Index"=w530:i32, "Plot Number"=w531:i32, "Message"=w524:string, "Removed?"=w532:bool)  [unwired: 3 in, 1 out]
      n157 = case shown="True" w532 {
        tunnel: w531 -> [_ w542]
        tunnel: w530 -> [_ w541]
        tunnel: w526 -> [w538 w540]
        tunnel: [w538 w539] -> w527
        frame False {
        }
        frame True {
          n158 = in-place {
            in-place-border: w542 -> [w546]
            in-place-border: w541 -> [w545]
            n159 = in-place-dvr #5(w540) -> (w544:T37)  [unwired: 1 out]
            n160 = in-place {
              in-place-border: w546 -> [w550]
              in-place-border: w545 -> [w548]
              n161 = in-place-cluster #6(w544) -> ("[Phasor Graph:Raw Phasor Plots]"=w547:T55[])
              n162 = Decrement(x=w550) -> (x-1=w549:i32)
              n163 = call "AlliGator Manage Phasor Plots Array.vi"("[Raw Phasor Plot] in"=w547, "Plot Index (-1: Last)"=w549, "Phasor Index(-1: Last)"=w548, "[Raw Phasor Plot] Action"=AlliGator_Raw_Phasor_Plot_Array_Action."Remove Phasor in Plot") -> ("[Raw Phasor Plot] out"=w552:T55[])  [unwired: 15 in]
              n164 = in-place-cluster #6("[Phasor Graph:Raw Phasor Plots]"=w552) -> (w543:T37)
            }
            n165 = in-place-dvr #5(w543) -> (w539:refnum<data-value>)  [unwired: 1 out]
          }
        }
      }
    }
    frame "Phasor Graph:Save All Phasor Plots" {
      # "\"Save All Phasor Plots\""
      n166 = call-poly "Variant to Data.vi"("Variant"=w572) -> ("Value"=w571:bool)  [unwired: 8 in]
      n167 = Unbundle By Name(w566) -> ("Registered Events Ctrl Refnums.Phasor Graph"=w567:refnum<vi>)
      n168 = call "AlliGator IV [Raw Phasor Plot].vi"("Get (F)/ Set (T)"=FALSE, "AlliGator IV DVR in"=w565) -> ("error out"=w562:errorcluster, "[Raw Phasor Plots]"=w563:T55[], "AlliGator IV DVR out"=w564:refnum<data-value>)  [unwired: 7 in]
      n169 = Not(x=w571) -> (.not. x?=w570:bool)
      n170 = call "Show Animated Busy Icon with Message.vi"("Already active? (F)"=w554, "Message"=w553, "Error In"=w562, "Target VI Refnum"=w555) -> ("Error Out"=w557:errorcluster)  [unwired: 7 in]
      n171 = for {
        tunnel: w563 -> [w582] mode=indexing
        tunnel: w567 -> [w581]
        tunnel: w570 -> [w578]
        tunnel: [w576] -> w569 mode=indexing
        tunnel: w557 -> [w575]
        tunnel: [w574] -> w560 mode=indexing
        i -> [w580]
        w577 = TRUE  # Save as...
        n172 = Increment(x=w580) -> (x+1=w579:i32)
        n173 = call "AlliGator Save Raw Phasor v2.vi"("Save only if selected"=w578, "Save as..."=w577, "error in (no error)"=w575, "Raw Phasor Plot"=w582, "Selected Plot"=w579, "Phasor Graph"=w581) -> ("Error Out"=w576:errorcluster, "Message"=w574:string)  [unwired: 4 in]
      }
      n174 = Merge Errors(w569) -> (w568:errorcluster)
      n175 = call "Hide Animated Busy Icon with Message.vi"("Already active? (F)"=w554, "Error In"=w568, "Target VI reference"=w555) -> ("Error Out"=w556:errorcluster)  [unwired: 8 in]
      n176 = call "Concatenate String Array.vi"("Separator (TAB)"="\r\n", "String Array"=w560) -> ("Formatted String"=w558:string)  [unwired: 9 in]
    }
    frame "Phasor Graph:Save Phasor Graph Image" {
      # "\"   Image\""
      n177 = call "AlliGator IV Dataset Path.vi"("Get (F)/ Set (T)"=FALSE, "error in (no error)"=w590, "AlliGator IV DVR in"=w601) -> ("error out"=w588:errorcluster, "[Time-Series Path]"=w598:path[], "Single Data Point Path"=w599:path, "AlliGator IV DVR out"=w600:refnum<data-value>, "Current Dataset"=w597:i32)  [unwired: 4 in]
      n178 = call "AlliGator Get Image File Format.vi"("Error In"=w590) -> ("error out"=w593:errorcluster, "File Extension (.xxx)"=w604:string, "Image File Format"=w603:T81)  [unwired: 7 in, 1 out]
      n179 = Unbundle By Name(w602) -> ("Registered Events Ctrl Refnums.Phasor Graph"=w605:refnum<vi>)
      n180 = call "Show Animated Busy Icon with Message.vi"("Already active? (F)"=w583, "Message"=w585, "Error In"=w588, "Target VI Refnum"=w584) -> ("Error Out"=w587:errorcluster)  [unwired: 7 in]
      n181 = Merge Errors(w587, w593) -> (w589:errorcluster)
      n182 = call "AlliGator Get Image Destination File Path.vi"("Image File Extension"=w604, "Image Name Prefix"="Phasor Graph " ("string"), "Error In"=w589, "Current Data Set"=w597, "Time-Series Paths"=w598, "Single Data Point Path"=w599) -> ("Error Out"=w592:errorcluster, "Image File Path"=w607:path)  [unwired: 4 in]
      n183 = call "XY Graph Save Graph Image.vi"("Error In"=w592, "Saved Image File Format"=w603, "Image File Path in"=w607, "XYGraph in"=w605) -> ("Error Out"=w594:errorcluster, "Image File Path out"=w606:path)  [unwired: 6 in]
      n184 = Path To String(path=w606) -> (string=w595:string)
      n185 = call "Hide Animated Busy Icon with Message.vi"("Already active? (F)"=w583, "Error In"=w594, "Target VI reference"=w584) -> ("Error Out"=w586:errorcluster)  [unwired: 8 in]
    }
    frame "Phasor Graph:Save Single Phasor Plot" {
      # "\"Save Phasor Plot\""
      n186 = Variant To Data(type=T31 {"Mouse Click Event Data"={"Multiplot XY Graph"=refnum, "Mouse Coordinates"={"Horizontal"=0, "Vertical"=0}}, "Save as..."=FALSE} ("output cluster"), Variant=w629) -> (data=w628:T31, error out=w614:errorcluster)  [unwired: 1 in]
      n187 = Unbundle(w628) -> ("Mouse Click Event Data"=w627:T20, "Save as..."=w621:bool)
      n188 = call "AlliGator IV [Raw Phasor Plot].vi"("Get (F)/ Set (T)"=FALSE, "error in (no error)"=w614, "AlliGator IV DVR in"=w617) -> ("error out"=w613:errorcluster, "[Raw Phasor Plots]"=w616:T55[], "AlliGator IV DVR out"=w618:refnum<data-value>)  [unwired: 6 in]
      n189 = Unbundle(w627) -> ("Multiplot XY Graph"=w623:T18, "Mouse Coordinates"=w622:T19)
      n190 = call-poly "Get Plot at Mouse Click.vi"("error in (no error)"=w613, "Mouse Click Coordinates"=w622, "XY Graph in"=w623) -> ("error out"=w626:errorcluster, "Plot at Coordinates"=w620:i32, "XY Graph out"=w625:T18)  [unwired: 2 in, 4 out]
      n191 = case shown="-1, 1, Default" w620 {
        selector: w620 -> [_ w641]
        tunnel: w626 -> [w631 w649]
        tunnel: w625 -> [_ w650]
        tunnel: w621 -> [_ w648]
        tunnel: w616 -> [_ w640]
        tunnel: [w631 w635] -> w619
        tunnel: [_ w637] -> w612
        tunnel: w611 -> [_ w634]
        tunnel: w610 -> [_ w633]
        tunnel: w609 -> [_ w632]
        frame 0 {
          # "UC"
        }
        frame -1, 1, Default {
          # "UC is not part of Z plot array"
          n192 = call "Show Animated Busy Icon with Message.vi"("Already active? (F)"=w632, "Message"=w634, "Error In"=w649, "Target VI Refnum"=w633) -> ("Error Out"=w636:errorcluster)  [unwired: 7 in]
          n193 = Array Size(array=w640) -> (size(s)=w639:i32)
          n194 = Less Than 0?(x=w641) -> (x < 0?=w642:bool)
          n195 = Decrement(x=w641) -> (x-1=w643:i32)
          n196 = Select(t=w641, s=w642, f=w643) -> (s? t:f=w644:i32)
          n197 = Select(t=w639, s=w642, f=w641) -> (s? t:f=w638:i32)
          n198 = call "(Signed) Index 1D Array.vim"("Signed Index"=w644, "Array"=w640) -> ("Array Element"=w645:T55)  [unwired: 9 in]
          n199 = call "AlliGator Script Destination File Path.vi"() -> ("Destination File Path"=w647:path)
          n200 = call "AlliGator Save Raw Phasor v2.vi"("Save as..."=w648, "Phasor Plot Path (empty)"=w647, "error in (no error)"=w636, "Raw Phasor Plot"=w645, "Selected Plot"=w638, "Phasor Graph"=w650) -> ("Error Out"=w646:errorcluster, "Message"=w637:string)  [unwired: 4 in]
          n201 = call "Hide Animated Busy Icon with Message.vi"("Already active? (F)"=w632, "Error In"=w646, "Target VI reference"=w633) -> ("Error Out"=w635:errorcluster)  [unwired: 8 in]
        }
      }
    }
    frame "Phasor Graph:Set Cursor n Location" {
      # "Set Cursor n Location"
      n202 = Variant To Data(type=T34 {"Current Phasor (g, s)"={"g"=0.0, "s"=0.0}, "Cursor Id"=0} ("output cluster"), Variant=w664) -> (data=w662:T34, error out=w660:errorcluster)  [unwired: 1 in]
      n203 = Unbundle By Name(w662) -> ("Cursor Id"=w657:u32, "Current Phasor (g, s)"=w661:T22)
      n204 = Unbundle By Name(w653) -> ("Registered Events Ctrl Refnums.Phasor Graph"=w654:refnum<vi>)
      n205 = Format Into String(format string=" (n = %d)", w657) -> (resulting string=w651:string)  [unwired: 2 in, 1 out]
      n206 = Decrement(x=w657) -> (x-1=w659:u32)
      n207 = property class="XYGraph (strict)"(reference=w654, error in=w660, "Active Cursor"=w659, "Cursor.Cursor Position"=w661) -> (error out=w655:errorcluster)  [unwired: 1 out]
    }
    frame "Phasor Graph:Set Reference n to Current Phase Lifetime Value" {
      # "\"Phasor Graph:Set Reference n to Current Phase Lifetime Value\""
      n208 = Unbundle By Name(w671) -> ("Phasor Graph Ctrl Refnums.Phase Lifetime"=w670:refnum<vi>)
      n209 = call-poly "Variant to Data.vi"("Variant"=w680) -> ("Value"=w673:i32)  [unwired: 8 in]
      n210 = property class="DigNum (strict)"(reference=w670) -> (error out=w668:errorcluster, "Value"=w669:dbl[unit])  [unwired: 1 in, 1 out]
      n211 = Format Into String(format string=" (n = %d)", w673) -> (resulting string=w667:string)  [unwired: 2 in, 1 out]
      n212 = case shown="No Error" w668 {
        tunnel: w679 -> [w699 w700]
        tunnel: [w698 w700] -> w678
        tunnel: w669 -> [w694 _]
        tunnel: w675 -> [w693 _]
        tunnel: [w692 _] -> w674
        tunnel: w673 -> [w683 _]
        frame No Error {
          n213 = call "Phasor Convert (tau, f) to (g, s) & (m, phi).vi"("Phasor Frequency"=w693, "Phase Lifetime"=w694) -> ("Error Out"=w692:errorcluster, "Phasor (g, s)"=w691:T22)  [unwired: 7 in, 1 out]
          n214 = Bundle("Phasor (g, s)"=w691, "Value"=w683) -> (w687:cluster{"Phasor (g, s)":T22, "Value":i32})  [unwired: 1 in]
          n215 = Build Array(w691) -> (w681:T22[])
          n216 = Bundle By Name(cluster=T35 {"Data Type"="Phasor Value", "Data"=variant} ("Phasor Reference Data"), "Data"=w687) -> (w685:T35)
          n217 = Bundle By Name(cluster=T6 {"AlliGator Q Event"=enum."Phasor Graph:Update Last Phasor Value", "Data"=variant} ("Alligator Atomic Action"), "Data"=w681) -> (w695:T6)
          n218 = Bundle By Name(cluster=T6 {"AlliGator Q Event"=enum."Phasor Ratio:Send Reference n to Notebook", "Data"=variant} ("Alligator Atomic Action"), "Data"=w683) -> (w682:T6)
          n219 = Bundle By Name(cluster=T6 {"AlliGator Q Event"=enum."Phasor Ratio:Use as Reference n", "Data"=variant} ("Alligator Atomic Action"), "Data"=w685) -> (w688:T6)
          n220 = Build Array(w695, w688, w682) -> (w689:T6[])
          n221 = call-poly "AlliGator Add Action(s) to Stack.vi"("Elements Order in Action Stack (Default: 2 BEFORE 1)"=Alligator_Elements_Order_in_Action_Stack."Enqueue 2 BEFORE 1", "Alligator Queue Element 2"=w689, "Alligator Queue Element 1"=w699) -> ("Alligator Queue Element 1 (+ 2)"=w698:T6[])  [unwired: 7 in, 1 out]
        }
        frame Error {
        }
      }
    }
    frame "Phasor Graph:Set Reference n to Lifetime Value" {
      # "Set Reference n to Lifetime Value"
      n222 = call-poly "Variant to Data.vi"("Variant"=w713) -> ("Value"=w704:i32)  [unwired: 8 in]
      n223 = Format Into String(format string=" (n = %d)", w704) -> (resulting string=w702:string)  [unwired: 2 in, 1 out]
      n224 = call "AlliGator Enter Reference Lifetime Dialog.vi"() -> ("Cancelled?"=w708:bool, "Reference Lifetime"=w707:dbl[unit])  [unwired: 9 in, 1 out]
      n225 = case shown="False" w708 {
        tunnel: w712 -> [w732 w733]
        tunnel: [w731 w733] -> w711
        tunnel: w707 -> [w727 _]
        tunnel: w706 -> [w726 _]
        tunnel: [w725 _] -> w705
        tunnel: w704 -> [w716 _]
        frame False {
          n226 = call "Phasor Convert (tau, f) to (g, s) & (m, phi).vi"("Phasor Frequency"=w726, "Phase Lifetime"=w727) -> ("Error Out"=w725:errorcluster, "Phasor (g, s)"=w724:T22)  [unwired: 7 in, 1 out]
          n227 = Bundle("Phasor (g, s)"=w724, "Value"=w716) -> (w720:cluster{"Phasor (g, s)":T22, "Value":i32})  [unwired: 1 in]
          n228 = Build Array(w724) -> (w714:T22[])
          n229 = Bundle By Name(cluster=T35 {"Data Type"="Phasor Value", "Data"=variant} ("Phasor Reference Data"), "Data"=w720) -> (w718:T35)
          n230 = Bundle By Name(cluster=T6 {"AlliGator Q Event"=enum."Phasor Graph:Update Last Phasor Value", "Data"=variant} ("Alligator Atomic Action"), "Data"=w714) -> (w728:T6)
          n231 = Bundle By Name(cluster=T6 {"AlliGator Q Event"=enum."Phasor Ratio:Send Reference n to Notebook", "Data"=variant} ("Alligator Atomic Action"), "Data"=w716) -> (w715:T6)
          n232 = Bundle By Name(cluster=T6 {"AlliGator Q Event"=enum."Phasor Ratio:Use as Reference n", "Data"=variant} ("Alligator Atomic Action"), "Data"=w718) -> (w721:T6)
          n233 = Build Array(w728, w721, w715) -> (w722:T6[])
          n234 = call-poly "AlliGator Add Action(s) to Stack.vi"("Elements Order in Action Stack (Default: 2 BEFORE 1)"=Alligator_Elements_Order_in_Action_Stack."Enqueue 2 BEFORE 1", "Alligator Queue Element 2"=w722, "Alligator Queue Element 1"=w732) -> ("Alligator Queue Element 1 (+ 2)"=w731:T6[])  [unwired: 7 in, 1 out]
        }
        frame True {
        }
      }
    }
    frame "Phasor Graph:Show Single Phasor" {
      # "\"Show Single Phasor\""
      n235 = Unbundle By Name(w740) -> ("Registered Events Ctrl Refnums.Phasor Graph"=w741:refnum<vi>)
      n236 = call "AlliGator IV Phasor Plot.vi"("Get (F)/ Set (T)"=FALSE, "AlliGator IV DVR in"=w739) -> ("Phasor Plot"=w737:cluster{"g Array":dbl[], "s Array":dbl[]}, "AlliGator IV DVR out"=w738:refnum<data-value>)  [unwired: 7 in, 1 out]
      n237 = call-poly "Variant to Data.vi"("Variant"=w748) -> ("Value"=w747:i32)  [unwired: 8 in]
      n238 = case shown="0, Default" w747 {
        selector: w747 -> [_ w782]
        tunnel: [w750 w779] -> w746
        tunnel: [w751 w769] -> w744
        tunnel: w737 -> [w750 w773]
        tunnel: w735 -> [w749 w772]
        tunnel: [w749 w771] -> w734
        frame ..-1 {
          # "Show the whole phasor plot"
          n239 = xnode "Error Ring"() -> ("error out"=w754:errorcluster)
          n240 = Unbundle By Name(w750) -> ("g Array"=w752:dbl[])
          n241 = xnode "Error Ring"() -> ("error out"=w753:errorcluster)
          n242 = Empty Array?(array=w752) -> (empty?=w755:bool)
          n243 = Select(t=w754, s=w755, f=w753) -> (s? t:f=w751:errorcluster)
        }
        frame 0, Default {
          n244 = Unbundle By Name(w773) -> ("g Array"=w777:dbl[], "s Array"=w783:dbl[])
          n245 = Decrement(x=w782) -> (x-1=w778:i32)
          n246 = xnode "Error Ring"() -> ("error out"=w775:errorcluster)
          n247 = Index Array(array=w777, index=w778) -> (element=w765:dbl)
          n248 = Index Array(array=w783, index=w778) -> (element=w764:dbl)
          n249 = Bundle By Name(cluster=T22 {"g"=0.0, "s"=0.0} ("Phasor"), "g"=w765, "s"=w764) -> (w762:T22)
          n250 = xnode "Error Ring"() -> ("error out"=w774:errorcluster)
          n251 = Build Array(w762) -> (w761:T22[])
          n252 = Build Array(w765) -> (w781:dbl[])
          n253 = Empty Array?(array=w777) -> (empty?=w776:bool)
          n254 = Build Array(w764) -> (w780:dbl[])
          n255 = Bundle By Name(cluster=T6 {"AlliGator Q Event"=enum."Phasor Graph:Update Last Phasor Value", "Data"=variant} ("Alligator Atomic Action"), "Data"=w761) -> (w766:T6)
          n256 = Select(t=w775, s=w776, f=w774) -> (s? t:f=w770:errorcluster)
          n257 = Bundle(w781, w780) -> (w779:cluster{dbl[], dbl[]})  [unwired: 1 in]
          n258 = call-poly "AlliGator Add Action(s) to Stack.vi"("Elements Order in Action Stack (Default: 2 BEFORE 1)"=Alligator_Elements_Order_in_Action_Stack."Enqueue 2 BEFORE 1", "Error In"=w770, "Alligator Atomic Action"=w766, "Alligator Queue Element 1"=w772) -> ("Error Out"=w769:errorcluster, "Alligator Queue Element 1 (+ 2)"=w771:T6[])  [unwired: 6 in]
        }
      }
      n259 = call "XY Graph Insert Plot.vi"("Error In"=w744, "Plot Index (Default Inf: Append to End)"=-1, "New Plot"=w746, "Multiplot XY Graph Refnum in"=w741) -> ("Error Out"=w742:errorcluster)  [unwired: 5 in, 2 out]
    }
    frame "Phasor Graph:Update Last Phasor Value" {
      w789 = TRUE ("Get (F)/ Set (T)")
      # "\"Update Last Phasor Value\""
      n260 = Unbundle By Name(w801) -> ("Phasor Graph Ctrl Refnums"=w800:T11)
      n261 = Variant To Data(type=T22[] [] ("Phasor"), Variant=w806) -> (data=w798:T22[], error out=w802:errorcluster)  [unwired: 1 in]
      n262 = Index Array(array=w798) -> (element #1=w796:T22, element #2=w790:T22)  [unwired: 2 in]
      n263 = call "AlliGator Update Phasor Graph Information at Cursor.vi"("Valid?"=TRUE, "Error In"=w802, "Phasor SDV"=w790, "Phasor"=w796, "Current Phasor Information Indicators"=w800) -> ("Error Out"=w797:errorcluster)  [unwired: 5 in, 1 out]
      n264 = call "AlliGator IV Last Calibrated Phasor.vi"("Get (F)/ Set (T)"=w789, "error in (no error)"=w797, "Last Calibrated Phasor"=w796, "AlliGator IV DVR in"=w799) -> ("error out"=w792:errorcluster, "AlliGator IV DVR out"=w794:refnum<data-value>)  [unwired: 5 in, 1 out]
      n265 = call "AlliGator IV Last Calibrated Phasor SDV.vi"("Get (F)/ Set (T)"=w789, "error in (no error)"=w792, "Last Calibrated Phasor SDV"=w790, "AlliGator IV DVR in"=w794) -> ("error out"=w791:errorcluster, "AlliGator IV DVR out"=w793:refnum<data-value>)  [unwired: 5 in, 1 out]
    }
    frame "Phasor Graph:Update Phasor (m, phi)" {
      # "\"Updated Phasor (m, phi)\""
      n266 = Unbundle By Name(w815) -> ("Phasor Graph Ctrl Refnums"=w814:T11)
      n267 = Variant To Data(type=T36 {"m"=0.0, "phi"=0.0} ("Phasor"), Variant=w821) -> (data=w818:T36, error out=w816:errorcluster)  [unwired: 1 in]
      n268 = call "Phasor Convert (m, phi) to (g,s).vi"("Phasor (m, phi)"=w818) -> ("Phasor (g, s)"=w811:T22)  [unwired: 8 in]
      n269 = call "AlliGator Update Phasor Graph Information at Cursor.vi"("Valid?"=TRUE, "Error In"=w816, "Phasor"=w811, "Current Phasor Information Indicators"=w814) -> ("Error Out"=w810:errorcluster)  [unwired: 6 in, 1 out]
      n270 = call "AlliGator IV Last Calibrated Phasor.vi"("Get (F)/ Set (T)"=TRUE, "error in (no error)"=w810, "Last Calibrated Phasor"=w811, "AlliGator IV DVR in"=w812) -> ("error out"=w809:errorcluster, "AlliGator IV DVR out"=w813:refnum<data-value>)  [unwired: 5 in, 1 out]
    }
    frame "Phasor Graph:Update SEPL Plot" {
      w825 = i32[] [5001, 5025, 5026]  # Not a Valid Plot, Incompatible References
      # "\"Update SEPL Plot\""
      n271 = call "Show Animated Busy Icon with Message.vi"("Already active? (F)"=w824, "Message"=w822, "Error In"=w823, "Target VI Refnum"=w827) -> ("Error Out"=w839:errorcluster)  [unwired: 7 in]
      n272 = Unbundle By Name(w829) -> ("Other AlliGator Ctrl Refnums.State Indicators"=w828:refnum<vi>, "Registered Events Ctrl Refnums.Phasor Graph"=w836:refnum<vi>)
      n273 = call "AlliGator Compute SEPL Plot.vi"("Error In"=w839) -> ("error out"=w841:errorcluster, "SEPL Plot"=w843:cluster{"X Array":dbl[], "Y Array":dbl[]}, "Plot Name"=w840:string)  [unwired: 7 in, 1 out]
      n274 = call "XY Graph Update Plot.vi"("New Plot Name (Default: unchanged)"=w840, "Error In"=w841, "Plot"=w843, "Plot Idx"=0 ("Plot Index (Default Inf: Append to End)"), "XY Graph refnum"=w836) -> ("Error Out"=w834:errorcluster)  [unwired: 6 in]
      n275 = call "AlliGator Get Updated Phasor Ratio References.vi"("error in (no error)"=w834) -> ("error out"=w831:errorcluster, "Phasor Ratio Reference 2"=w832:T22, "Phasor Ratio Reference 1"=w833:T22)  [unwired: 8 in]
      n276 = call "AlliGator Define Phasor References.vi"("Phasor Graph"=w836, "State Indicators Refnum"=w828, "Phasor 1"=w833, "Phasor 2"=w832, "Phasor Frequency"=w835, "Error In"=w831) -> ("Error Out"=w837:errorcluster)  [unwired: 5 in, 4 out]
      n277 = call "Hide Animated Busy Icon with Message.vi"("Already active? (F)"=w824, "Error In"=w837, "Target VI reference"=w827) -> ("Error Out"=w838:errorcluster)  [unwired: 8 in]
      n278 = call "Filter Errors.vi"("Filtered Errors"=w825, "error in (no error)"=w838) -> ("error out"=w830:errorcluster)  [unwired: 7 in]
    }
    frame "Phasor Graph:Use Cursor n Location" {
      # "Cursor #"
      # "\"Use Cursor n Location\""
      n279 = call-poly "Variant to Data.vi"("Variant"=w861) -> ("Value"=w853:u32)  [unwired: 8 in]
      n280 = Format Into String(format string=" (n = %d)", w853) -> (resulting string=w845:string)  [unwired: 2 in, 1 out]
      n281 = Unbundle By Name(w848) -> ("Registered Events Ctrl Refnums.Phasor Graph"=w849:refnum<vi>)
      n282 = Decrement(x=w853) -> (x-1=w854:u32)
      n283 = property class="XYGraph (strict)"(reference=w849, "Active Cursor"=w854) -> (error out=w850:errorcluster, "Cursor.Cursor Position"=w855:T82)  [unwired: 1 in, 1 out]
      n284 = Build Array(w855) -> (w846:T82[])
      n285 = Bundle By Name(cluster=T6 {"AlliGator Q Event"=enum."Phasor Graph:Update Last Phasor Value", "Data"=variant} ("Alligator Atomic Action"), "Data"=w846) -> (w856:T6)
      n286 = call-poly "AlliGator Add Action(s) to Stack.vi"("Elements Order in Action Stack (Default: 2 BEFORE 1)"=Alligator_Elements_Order_in_Action_Stack."Enqueue 2 BEFORE 1", "Alligator Atomic Action"=w856, "Alligator Queue Element 1"=w860) -> ("Alligator Queue Element 1 (+ 2)"=w859:T6[])  [unwired: 7 in, 1 out]
    }
    frame "Phasor Graph:Use Selected Plots Fitted Line/UC Intersections" {
      # "\"Phasor Graph: Use Selected Plots Fitted Line/UC Intersections\""
      n287 = Variant To Data(type=T18 refnum ("Multiplot XY Graph"), Variant=w899) -> (data=w886:T18, error out=w885:errorcluster)  [unwired: 1 in]
      n288 = Unbundle By Name(w876) -> ("Other AlliGator Ctrl Refnums.State Indicators"=w888:refnum<vi>, "Phasor Graph Ctrl Refnums.Phase Lifetime 1"=w875:refnum<vi>, "Phasor Graph Ctrl Refnums.Phase Lifetime 2"=w874:refnum<vi>, "Phasor Graph Ctrl Refnums.Show Line"=w873:refnum<vi>)
      n289 = call "Show Animated Busy Icon with Message.vi"("Already active? (F)"=w864, "Error In"=w885, "Target VI Refnum"=w866) -> ("Error Out"=w868:errorcluster)  [unwired: 8 in]
      n290 = call "XY Graph Get Selected Plot Names & Indices.vi"("error in (no error)"=w868, "XY Graph in"=w886) -> ("error out"=w884:errorcluster, "Selected Plot Indices"=w879:i32[], "Selected Plot Names"=w883:string[])  [unwired: 5 in, 2 out]
      n291 = call-poly <userlib>:"Filter 1D Array__ogtk.vi"("items to filter"=0, "array"=w879) -> ("filtered array"=w878:i32[])  [unwired: 4 in, 1 out]
      n292 = call "Concatenate String Array.vi"("Separator (TAB)"=", ", "Suffix (\"\")"="):" ("Suffix (\"\")"), "String Array"=w883, "Prefix (\"\")"=" (" ("Prefix (\"\")")) -> ("Formatted String"=w863:string)  [unwired: 7 in]
      n293 = for {
        tunnel: [w905] -> w890 mode=concatenating
        tunnel: w886 -> [w903]
        tunnel: w884 -> [w902]
        tunnel: [w904] -> w889
        tunnel: w878 -> [w901] mode=indexing
        n294 = call "AlliGator Get Phasor Plot Data.vi"("error in (no error)"=w902, "Plot Idx (-1: last)"=w901, "Phasor Graph Refnum"=w903) -> ("error out"=w904:errorcluster, "Phasor Array"=w905:T22[])  [unwired: 5 in, 2 out]
      }
      n295 = call "Phasor Find Intersections of Fitted Line with Universal Circle.vi"("Error In"=w889, "Phasor Array"=w890) -> ("Error Out"=w892:errorcluster, "Intersection 2"=w893:T22, "Intersection 1"=w894:T22)  [unwired: 7 in]
      n296 = Unbundle By Name(w892) -> ("status"=w891:bool)
      n297 = call "AlliGator Define Phasor References.vi"("Phasor Graph"=w886, "State Indicators Refnum"=w888, "Phasor 1"=w894, "Phasor 2"=w893, "Phasor Frequency"=w869, "Error In"=w892) -> ("Reference Lifetime 1"=w898:dbl[unit], "Reference Lifetime 2"=w897:dbl[unit], "Phasor Reference 1"=w896:T22, "Phasor Reference 2"=w895:T22, "Error Out"=w872:errorcluster)  [unwired: 5 in]
      n298 = Not(x=w891) -> (.not. x?=w870:bool)
      n299 = call "Hide Animated Busy Icon with Message.vi"("Already active? (F)"=w864, "Error In"=w872, "Target VI reference"=w866) -> ("Error Out"=w867:errorcluster)  [unwired: 8 in]
      n300 = property class="Bool (strict)"(reference=w873, error in=w867, "Val(Sgnl)"=w870) -> (error out=w871:errorcluster)  [unwired: 1 out]
      n301 = case shown="No Error" w867 {
        tunnel: w898 -> [w908 _]
        tunnel: w897 -> [w907 _]
        tunnel: w896 -> [_ _]
        tunnel: w895 -> [_ _]
        tunnel: w875 -> [w910 _]
        tunnel: w874 -> [w909 _]
        frame No Error {
          w906 = TRUE ("Visible")
          n302 = property class="DigNum (strict)"(reference=w910, "Value"=w908, "Visible"=w906) -> ()  [unwired: 1 in, 2 out]
          n303 = property class="DigNum (strict)"(reference=w909, "Value"=w907, "Visible"=w906) -> ()  [unwired: 1 in, 2 out]
        }
        frame Error {
        }
      }
    }
    frame "Phasor Graph:Use Selected Plots Principal Axis/UC Intersections" {
      # "\"Phasor Graph: Use Selected Plots Principal Axis/UC Intersections\""
      n304 = call-poly "Variant to Data.vi"("Variant"=w932) -> ("Value"=w929:bool)  [unwired: 8 in]
      n305 = Unbundle By Name(w927) -> ("Registered Events Ctrl Refnums.Phasor Graph"=w920:refnum<vi>, "Phasor Graph Ctrl Refnums.Phase Lifetime 1"=w926:refnum<vi>, "Phasor Graph Ctrl Refnums.Phase Lifetime 2"=w925:refnum<vi>, "Other AlliGator Ctrl Refnums.State Indicators"=w919:refnum<vi>, "Phasor Graph Ctrl Refnums.Show Line"=w921:refnum<vi>)
      n306 = call "XY Graph Get Selected Plot Names & Indices.vi"("XY Graph in"=w920) -> ("error out"=w939:errorcluster, "Selected Plot Indices"=w931:i32[], "Selected Plot Names"=w938:string[], "XY Graph out"=w930:T18)  [unwired: 6 in, 1 out]
      n307 = call-poly <userlib>:"Filter 1D Array__ogtk.vi"("items to filter"=0, "array"=w931) -> ("filtered array"=w934:i32[])  [unwired: 4 in, 1 out]
      n308 = call "Concatenate String Array.vi"("Separator (TAB)"=", ", "Suffix (\"\")"="):" ("Suffix (\"\")"), "String Array"=w938, "Prefix (\"\")"=" (" ("Prefix (\"\")")) -> ("Formatted String"=w928:string)  [unwired: 7 in]
      n309 = call "Show Animated Busy Icon with Message.vi"("Already active? (F)"=w912, "Error In"=w939, "Target VI Refnum"=w915) -> ("Error Out"=w917:errorcluster)  [unwired: 8 in]
      n310 = call "AlliGator Use Phasor Graph Selected Phasor Plots Principal Axis - UC Intersections as References.vi"("Selected Plot List"=w928, "error in (no error)"=w917, "Major Axis?"=w929, "Selected Plot Indices"=w934, "Phasor Graph refnum"=w930) -> ("error out"=w941:errorcluster, "Message"=w913:string, "Intersection 1"=w943:cluster{"x":dbl, "y":dbl}, "Intersection 2"=w942:cluster{"x":dbl, "y":dbl})  [unwired: 3 in]
      n311 = call "Hide Animated Busy Icon with Message.vi"("Already active? (F)"=w912, "Error In"=w941, "Target VI reference"=w915) -> ("Error Out"=w916:errorcluster)  [unwired: 8 in]
      n312 = Unbundle By Name(w916) -> ("status"=w940:bool)
      n313 = call "AlliGator Define Phasor References.vi"("Phasor Graph"=w920, "State Indicators Refnum"=w919, "Phasor 1"=w943, "Phasor 2"=w942, "Phasor Frequency"=w918, "Error In"=w916) -> ("Reference Lifetime 1"=w947:dbl[unit], "Reference Lifetime 2"=w946:dbl[unit], "Phasor Reference 1"=w945:T22, "Phasor Reference 2"=w944:T22, "Error Out"=w923:errorcluster)  [unwired: 5 in]
      n314 = Not(x=w940) -> (.not. x?=w924:bool)
      n315 = case shown="No Error" w923 {
        tunnel: w947 -> [w952 _]
        tunnel: w946 -> [w950 _]
        tunnel: w945 -> [_ _]
        tunnel: w944 -> [_ _]
        tunnel: w926 -> [w953 _]
        tunnel: w925 -> [w951 _]
        frame No Error {
          w949 = TRUE ("Visible")
          n316 = property class="DigNum (strict)"(reference=w953, "Value"=w952, "Visible"=w949) -> ()  [unwired: 1 in, 2 out]
          n317 = property class="DigNum (strict)"(reference=w951, "Value"=w950, "Visible"=w949) -> ()  [unwired: 1 in, 2 out]
        }
        frame Error {
        }
      }
      n318 = property class="Bool (strict)"(reference=w921, error in=w923, "Val(Sgnl)"=w924) -> (error out=w922:errorcluster)  [unwired: 1 out]
    }
    frame "Phasor Graph:Use UC/Cursor-Defined Line Intersections" {
      w963 = TRUE ("Visible")
      # "Use UC/Cursor-Defined Line Intersections"
      n319 = Unbundle By Name(w966) -> ("Phasor Graph Ctrl Refnums.Phase Lifetime 1"=w970:refnum<vi>, "Phasor Graph Ctrl Refnums.Phase Lifetime 2"=w969:refnum<vi>, "Other AlliGator Ctrl Refnums.State Indicators"=w971:refnum<vi>, "Registered Events Ctrl Refnums.Phasor Graph"=w972:refnum<vi>)  [unwired: 1 out]
      n320 = Unbundle By Name(w966) -> ("Phasor Graph Ctrl Refnums.Phasor Reference 1 Control"=w965:refnum<vi>)
      n321 = call "Show Animated Busy Icon with Message.vi"("Already active? (F)"=w957, "Message"=w955, "Error In"=w960, "Target VI Refnum"=w956) -> ("Error Out"=w959:errorcluster)  [unwired: 7 in]
      n322 = call "AlliGator Find Cursor Connecting Line Intersection(s) with Universal Circle.vi"("Error In"=w959, "XY Graph Refnum"=w972) -> ("Error Out"=w975:errorcluster, "Intersection 2"=w976:cluster{"x":dbl, "y":dbl}, "Intersection 1"=w977:cluster{"x":dbl, "y":dbl})  [unwired: 7 in]
      n323 = call "AlliGator Define Phasor References.vi"("Phasor Graph"=w972, "State Indicators Refnum"=w971, "Phasor 1"=w977, "Phasor 2"=w976, "Phasor Frequency"=w973, "Error In"=w975) -> ("Reference Lifetime 1"=w968:dbl[unit], "Reference Lifetime 2"=w967:dbl[unit], "Error Out"=w961:errorcluster)  [unwired: 5 in, 2 out]
      n324 = call "Hide Animated Busy Icon with Message.vi"("Already active? (F)"=w957, "Error In"=w961, "Target VI reference"=w956) -> ("Error Out"=w958:errorcluster)  [unwired: 8 in]
      n325 = call "Phasor Convert (tau, f) to (m, phi).vi"("Lifetime"=w968, "Phasor Frequency"=w973) -> ("Phasor (m, phi)"=w974:T36)  [unwired: 5 in]
      n326 = Unbundle By Name(w974) -> ("phi"=w964:dbl)
      n327 = property class="DigNum (strict)"(reference=w970, "Value"=w968, "Visible"=w963) -> ()  [unwired: 1 in, 2 out]
      n328 = property class="DigNum (strict)"(reference=w969, "Value"=w967, "Visible"=w963) -> ()  [unwired: 1 in, 2 out]
      n329 = property class="Scroll (strict)"(reference=w965, "Value"=w964) -> ()  [unwired: 1 in, 2 out]
    }
  }
  "Data Value Reference out" <- w20
  "error out" <- w9
  "Script out" <- w12
  "AlliGator Q Elements out" <- w11
  n330 = call "Get Current Message Text Format.vi"("Text Format"=w1) -> ("Message Formatting"=w4:T2)  [unwired: 8 in, 1 out]
  n331 = call "AlliGator Package Notebook Messages.vi"("Message Formatting"=w4, "Message"=w3, "AlliGator Q Event in"="AlliGator Q Event in") -> ("[Notebook Message]"=→"[Notebook Message]":T1[])  [unwired: 8 in]
